vi "Parameter.vi"(9 "In":string, 10 "VIId":string, 11 "VariablesRef":T4) -> ()   [LabVIEW 2018, in "String.lvlib"]
uses:
  String.lvlib
  <userlib>/_OpenG.lib/dictionary/dictionary.llb/Dictionary Object RefNum__ogtk.ctl
  <userlib>/_OpenG.lib/dictionary/dictionary.llb/Dictionary Object RefNum - Enum__ogtk.ctl
  <vilib>/Utility/error.llb/whitespace.ctl
  <vilib>/addons/_JKI.lib/Serialization/JSON/JKI JSON Serialization.lvlib
panel:
  in  "Tab Control":enum32{"Config", "控件"}(tab)
  in  "ArrayType":T1(tab)
  in  "字符串_InitialString":string caption="字符串(可通过${..}调用组合字符串)"
  in  "长度_StringSubset":i32 caption="长度"
  in  "偏移_StringSubset":i32 caption="偏移"
  in  "位置_TrimWhitespace":T2 caption="位置" items=["both", "start of string", "end of string"]
  in  "长度_ReplaceSubstring":i32 caption="长度"
  in  "偏移_ReplaceSubstring":i32 caption="偏移"
  in  "子字符串_ReplaceSubstring":string caption="子字符串(可通过${..}调用组合字符串)"
  in  "IgnoreCase_SearchandReplaceString":bool caption="IgnoreCase"
  in  "ReplaceAll_SearchandReplaceString":bool caption="ReplaceAll"
  in  "替换字符串_SearchandReplaceString":string caption="替换字符串(可通过${..}调用组合字符串)"
  in  "偏移_SearchandReplaceString":i32 caption="偏移"
  in  "搜索字符串_SearchandReplaceString":string caption="搜索字符串(可通过${..}调用组合字符串)"
  in  "偏移_MatchPattern":i32 caption="偏移"
  in  "正则表达式_MatchPattern":string caption="正则表达式(仅支持部分正则)"
  in  "多行_MatchRegularExpression":bool caption="多行"
  in  "忽略大小写_MatchRegularExpression":bool caption="忽略大小写"
  in  "偏移_MatchRegularExpression":i32 caption="偏移"
  in  "正则表达式_MatchRegularExpression":string caption="正则表达式(支持全部正则)"
  in  "UTC格式_FormatDate/TimeString":bool
  in  "时间格式字符串_FormatDate/TimeString":string
  in  "忽略大小写_StartWith":bool caption="忽略大小写"
  in  "子字符串_StartWith":string caption="子字符串(可通过${..}调用组合字符串)"
  in  "子字符串_EndWith":string caption="子字符串(可通过${..}调用组合字符串)"
  in  "忽略大小写_EndWith":bool caption="忽略大小写"
  in  "SubString_AfterSubstring":string caption="子字符串(可通过${..}调用组合字符串)"
  in  "SubString_BeforeSubstring":string caption="子字符串(可通过${..}调用组合字符串)"
  in  "后子字符串_MiddleSubstring":string caption="后子字符串(可通过${..}调用组合字符串)"
  in  "前子字符串_MiddleSubstring":string caption="前子字符串(可通过${..}调用组合字符串)"
  in  "Delimiter_StringTo1DArray":string="\t"
  in  "字符串变量(StringVar)":u16(ring) items=["", "SN", "FileName", "ProductName", "TestLine", "TestStation"]
  in  "方法(Method)":T3(ring)
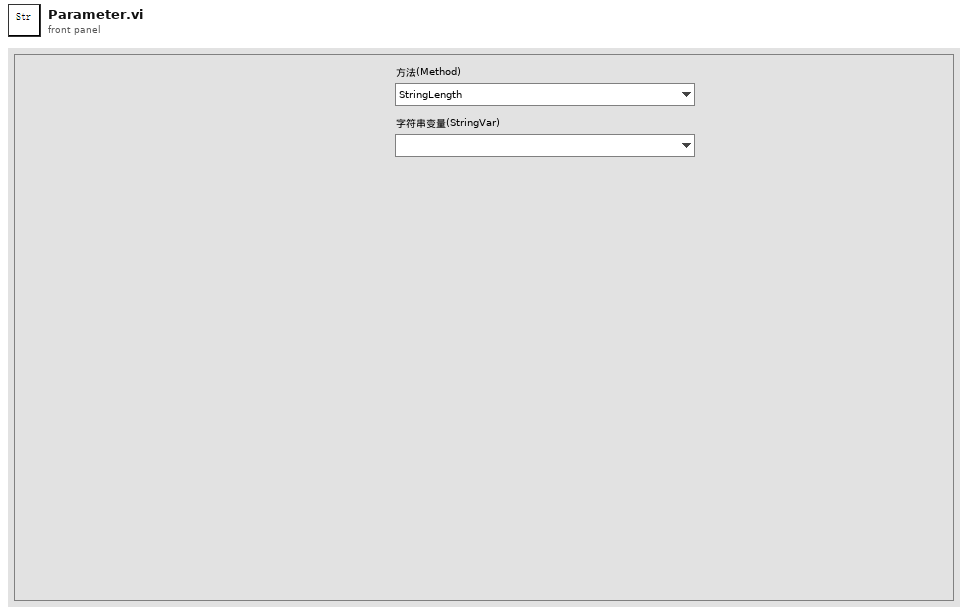
[diagram p1: front panel]
types:
  T1 = enum32{"StringLength", "InitialString", "StringSubset", "TrimWhitespace", "ReplaceSubstring", "SearchandReplaceString", "MatchPattern", "MatchRegularExpression", "FormatDate/TimeString", "ToLowerCase", "ToUpperCase", "StringMD5", "NumStringToHexString", "HexStringToNumString", "StartWith", "EndWith", "AfterSubstring", "BeforeSubstring", "MiddleSubstring", "AsciiToHexString", "HexStringToAscii", "StringTo1DArray", "StringToCharacterArray", "RemoveAllWhitespace"}
  T2 = typedef "whitespace.ctl" = u16
  T3 = enum16{"StringLength", "InitialString", "StringSubset", "TrimWhitespace", "ReplaceSubstring", "SearchandReplaceString", "MatchPattern", "MatchRegularExpression", "FormatDate/TimeString", "ToLowerCase", "ToUpperCase", "StringMD5", "NumStringToHexString", "HexStringToNumString", "StartWith", "EndWith", "AfterSubstring", "BeforeSubstring", "MiddleSubstring", "AsciiToHexString", "HexStringToAscii", "StringTo1DArray", "StringToCharacterArray", "RemoveAllWhitespace"}
  T4 = typedef "Dictionary Object RefNum__ogtk.ctl" = refnum<k1>
  T5 = cluster{"StringLength":cluster{"json":cluster{"Method":string, "StringVar":string}}, "InitialString":cluster{"json":cluster{"Method":string, "Strings":string}}, "StringSubset":cluster{"json":cluster{"Method":string, "StringVar":string, "offset":i32, "length":i32}}, "TrimWhitespace":cluster{"json":cluster{"Method":string, "StringVar":string, "Location":string}}, "ReplaceSubstring":cluster{"json":cluster{"Method":string, "StringVar":string, "Substring":string, "Offset":i32, "Length":i32}}, "SearchandReplaceString":cluster{"json":cluster{"Method":string, "StringVar":string, "SearchString":string, "Offset":i32, "ReplaceString":string, "ReplaceAll":bool, "IgnoreCase":bool}}, "MatchPattern":cluster{"json":cluster{"Method":string, "StringVar":string, "RegularExpression ":string, "Offset":i32}}, "MatchRegularExpression":cluster{"json":cluster{"Method":string, "StringVar":string, "RegularExpression ":string, "Offset":i32, "IgnoreCase":bool, "Multiline":bool}}, "FormatDate/TimeString":cluster{"json":cluster{"Method":string, "TimeFormatString ":string, "UTCFormat":bool}}, "ToLowerCase":cluster{"json":cluster{"Method":string, "StringVar":string}}, "ToUpperCase":cluster{"json":cluster{"Method":string, "StringVar":string}}, "StringMD5":cluster{"json":cluster{"Method":string, "StringVar":string}}, "NumStringToHexString":cluster{"json":cluster{"Method":string, "StringVar":string}}, "HexStringToNumString":cluster{"json":cluster{"Method":string, "StringVar":string}}, "StartWith":cluster{"json":cluster{"Method":string, "StringVar":string, "SubString":string, "IgnoreCasse":bool}}, "EndWith":cluster{"json":cluster{"Method":string, "StringVar":string, "SubString":string, "IgnoreCasse":bool}}, "AfterSubstring":cluster{"json":cluster{"Method":string, "StringVar":string, "SubString":string}}, "BeforeSubstring":cluster{"json":cluster{"Method":string, "StringVar":string, "SubString":string}}, "MiddleSubstring":cluster{"json":cluster{"Method":string, "StringVar":string, "BeforeSubString":string, "AfterSubString":string}}, "AsciiToHexString":cluster{"json":cluster{"Method":string, "StringVar":string}}, "HexStringToAscii":cluster{"json":cluster{"Method":string, "StringVar":string}}, "StringTo1DArray":cluster{"json":cluster{"Method":string, "StringVar":string, "Delimiter":string}}, "StringToCharacterArray":cluster{"json":cluster{"Method":string, "StringVar":string}}, "RemoveAllWhitespace":cluster{"json":cluster{"Method":string, "StringVar":string}}}
  T6 = enum32{"Invalid", "Standard", "Closed", "Hidden", "Minimized", "Maximized"}
  T7 = enum32{"invalid app kind", "Development System", "Run Time System", "Student Edition", "Embedded LabVIEW", "Evaluation", "Custom"}
  T8 = cluster{"Core":cluster{"Current VI Reference":refnum<vi>, "Close Panel on Exit?":bool}, "Parameter":cluster{"VariableRef":T4}, "Synchronize":cluster{"EnqueueData":cluster{"Action":enum16{"Create", "Query", "Revert", "UpdateVariable", "Close"}, "Data":variant}, "Echo":cluster{"VIRef":refnum<vi>, "JsonOut":string, "Status":string}, "Communicate":cluster{"ID":string, "JsonIn":string, "VarRef":T4}, "Queue":refnum<queue>}, "StringClusters":cluster{"StringLength":cluster{"json":cluster{"Method":string, "StringVar":string}}, "InitialString":cluster{"json":cluster{"Method":string, "Strings":string}}, "StringSubset":cluster{"json":cluster{"Method":string, "StringVar":string, "offset":i32, "length":i32}}, "TrimWhitespace":cluster{"json":cluster{"Method":string, "StringVar":string, "Location":string}}, "ReplaceSubstring":cluster{"json":cluster{"Method":string, "StringVar":string, "Substring":string, "Offset":i32, "Length":i32}}, "SearchandReplaceString":cluster{"json":cluster{"Method":string, "StringVar":string, "SearchString":string, "Offset":i32, "ReplaceString":string, "ReplaceAll":bool, "IgnoreCase":bool}}, "MatchPattern":cluster{"json":cluster{"Method":string, "StringVar":string, "RegularExpression ":string, "Offset":i32}}, "MatchRegularExpression":cluster{"json":cluster{"Method":string, "StringVar":string, "RegularExpression ":string, "Offset":i32, "IgnoreCase":bool, "Multiline":bool}}, "FormatDate/TimeString":cluster{"json":cluster{"Method":string, "TimeFormatString ":string, "UTCFormat":bool}}, "ToLowerCase":cluster{"json":cluster{"Method":string, "StringVar":string}}, "ToUpperCase":cluster{"json":cluster{"Method":string, "StringVar":string}}, "StringMD5":cluster{"json":cluster{"Method":string, "StringVar":string}}, "NumStringToHexString":cluster{"json":cluster{"Method":string, "StringVar":string}}, "HexStringToNumString":cluster{"json":cluster{"Method":string, "StringVar":string}}, "StartWith":cluster{"json":cluster{"Method":string, "StringVar":string, "SubString":string, "IgnoreCasse":bool}}, "EndWith":cluster{"json":cluster{"Method":string, "StringVar":string, "SubString":string, "IgnoreCasse":bool}}, "AfterSubstring":cluster{"json":cluster{"Method":string, "StringVar":string, "SubString":string}}, "BeforeSubstring":cluster{"json":cluster{"Method":string, "StringVar":string, "SubString":string}}, "MiddleSubstring":cluster{"json":cluster{"Method":string, "StringVar":string, "BeforeSubString":string, "AfterSubString":string}}, "AsciiToHexString":cluster{"json":cluster{"Method":string, "StringVar":string}}, "HexStringToAscii":cluster{"json":cluster{"Method":string, "StringVar":string}}, "StringTo1DArray":cluster{"json":cluster{"Method":string, "StringVar":string, "Delimiter":string}}, "StringToCharacterArray":cluster{"json":cluster{"Method":string, "StringVar":string}}, "RemoveAllWhitespace":cluster{"json":cluster{"Method":string, "StringVar":string}}}}
  T9 = cluster{"EnqueueData":cluster{"Action":enum16{"Create", "Query", "Revert", "UpdateVariable", "Close"}, "Data":variant}, "Echo":cluster{"VIRef":refnum<vi>, "JsonOut":string, "Status":string}, "Communicate":cluster{"ID":string, "JsonIn":string, "VarRef":T4}, "Queue":refnum<queue>}
  T10 = cluster{"Current VI Reference":refnum<vi>, "Close Panel on Exit?":bool}
  T11 = cluster{"json":cluster{"Method":string, "StringVar":string}}
  T12 = cluster{"json":cluster{"Method":string, "Strings":string}}
  T13 = cluster{"json":cluster{"Method":string, "StringVar":string, "offset":i32, "length":i32}}
  T14 = cluster{"json":cluster{"Method":string, "StringVar":string, "Location":string}}
  T15 = cluster{"json":cluster{"Method":string, "StringVar":string, "Substring":string, "Offset":i32, "Length":i32}}
  T16 = cluster{"json":cluster{"Method":string, "StringVar":string, "SearchString":string, "Offset":i32, "ReplaceString":string, "ReplaceAll":bool, "IgnoreCase":bool}}
  T17 = cluster{"json":cluster{"Method":string, "StringVar":string, "RegularExpression ":string, "Offset":i32}}
  T18 = cluster{"json":cluster{"Method":string, "StringVar":string, "RegularExpression ":string, "Offset":i32, "IgnoreCase":bool, "Multiline":bool}}
  T19 = cluster{"json":cluster{"Method":string, "TimeFormatString ":string, "UTCFormat":bool}}
  T20 = cluster{"json":cluster{"Method":string, "StringVar":string, "SubString":string, "IgnoreCasse":bool}}
  T21 = cluster{"json":cluster{"Method":string, "StringVar":string, "SubString":string}}
  T22 = cluster{"json":cluster{"Method":string, "StringVar":string, "BeforeSubString":string, "AfterSubString":string}}
  T23 = cluster{"json":cluster{"Method":string, "StringVar":string, "Delimiter":string}}
  T24 = cluster{"Action":enum16{"Create", "Query", "Revert", "UpdateVariable", "Close"}, "Data":variant}
  T25 = cluster{"ID":string, "JsonIn":string, "VarRef":T4}
  T26 = enum16{"Create", "Query", "Revert", "UpdateVariable", "Close"}
  T27 = cluster{"VIRef":refnum<vi>, "JsonOut":string, "Status":string}
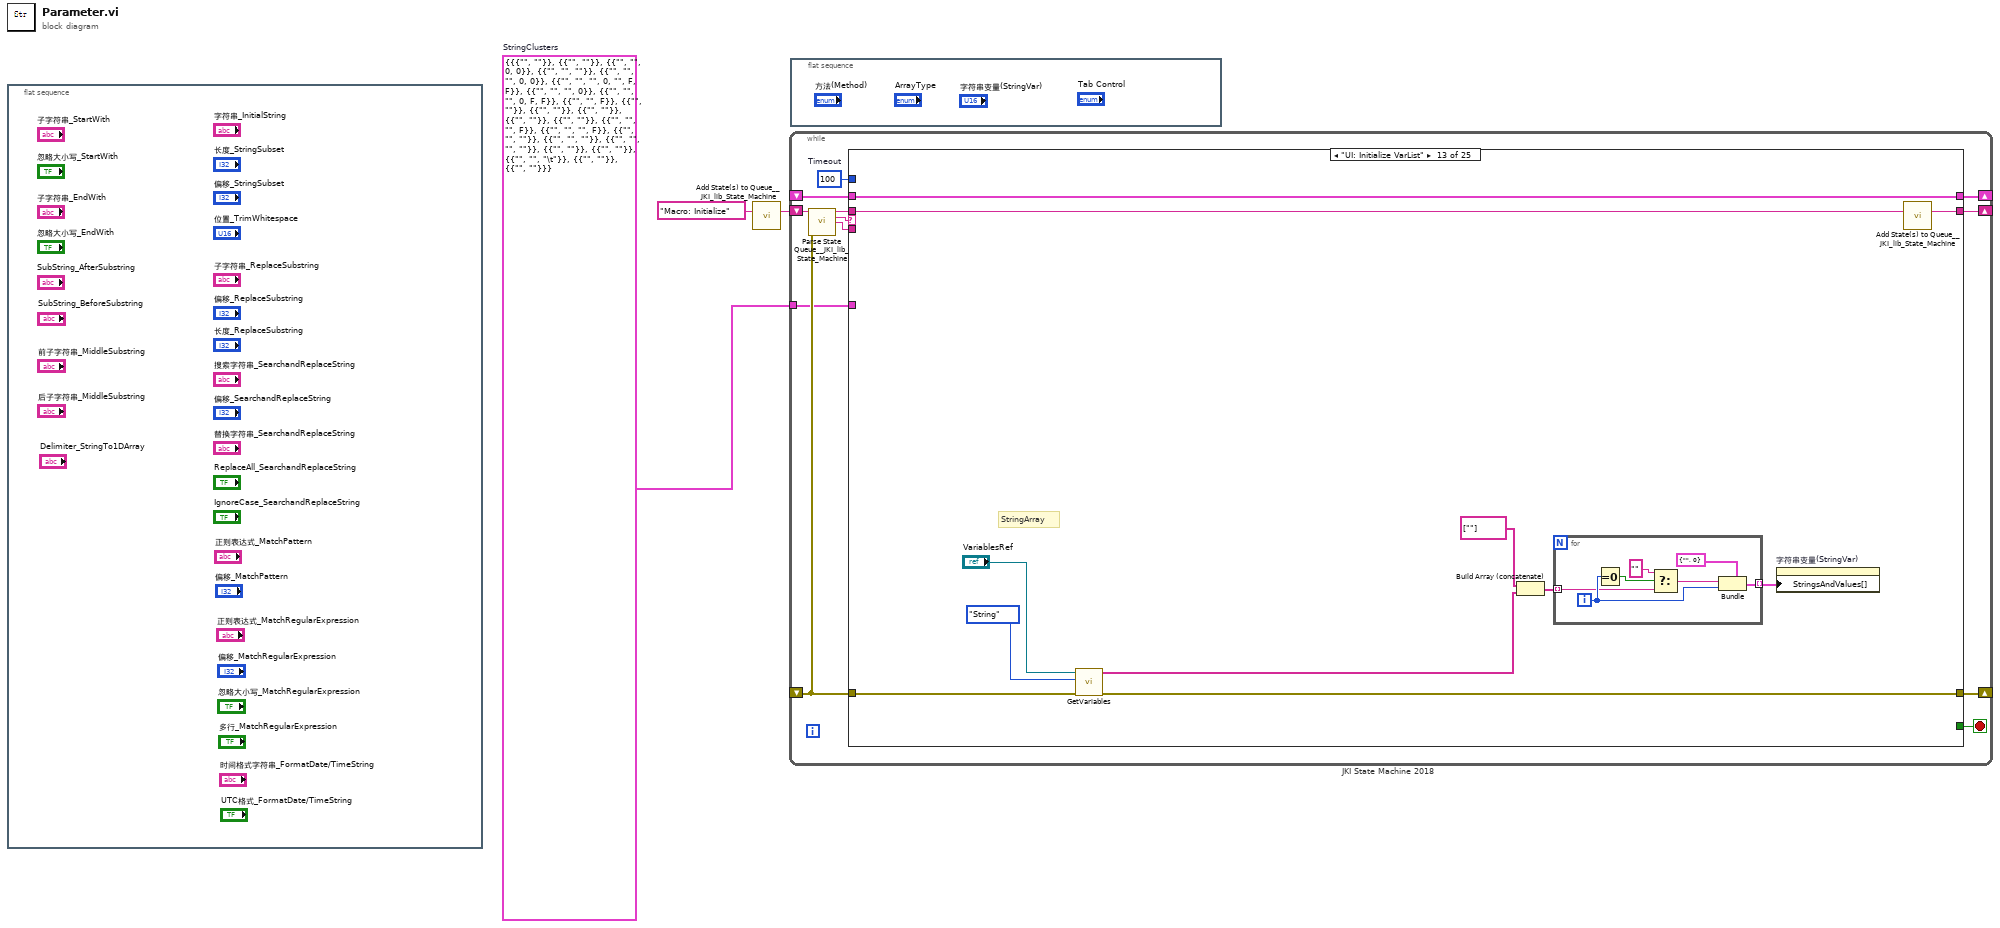
[diagram p0: block diagram]
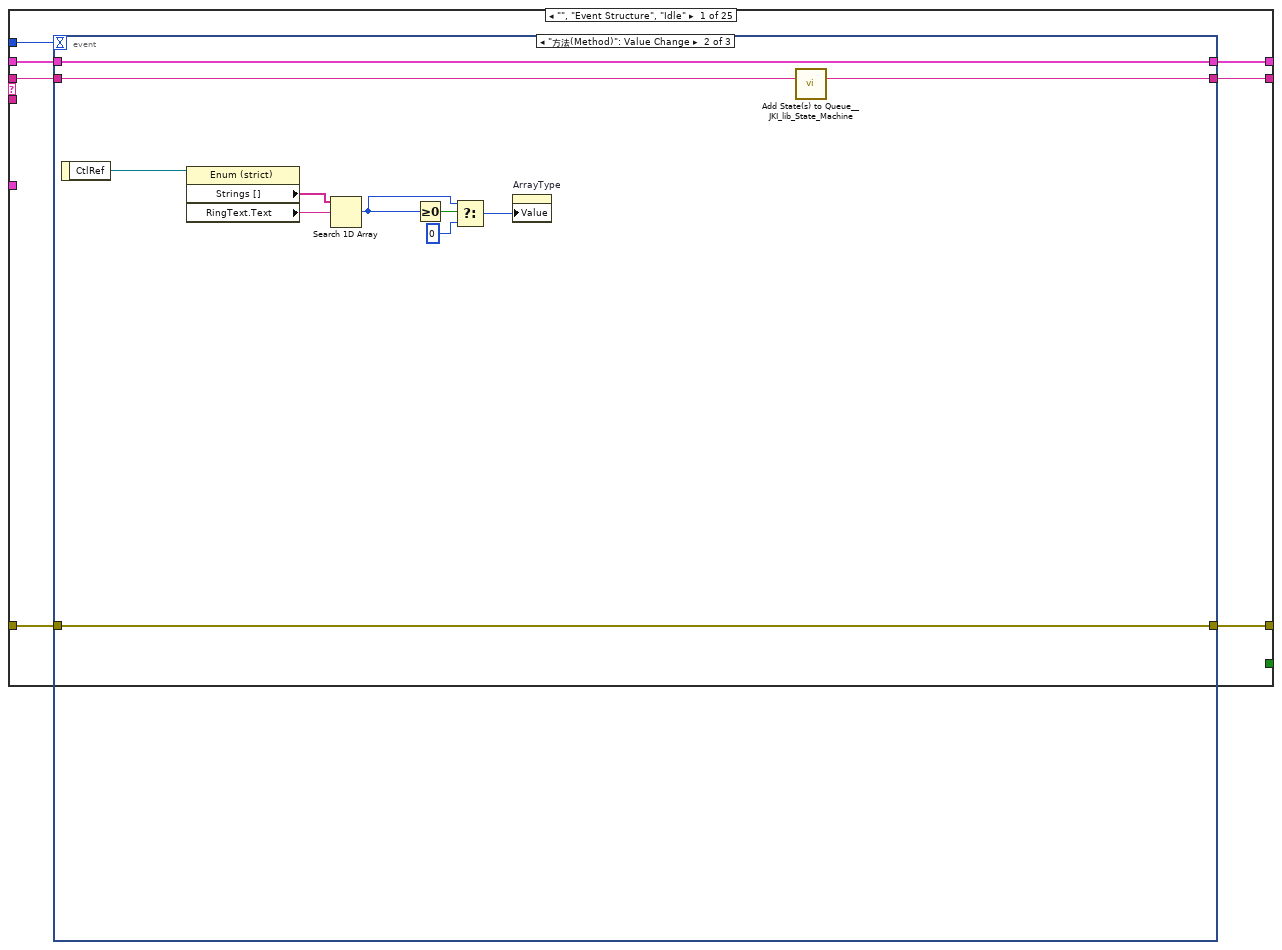
[diagram p2: hidden frame]
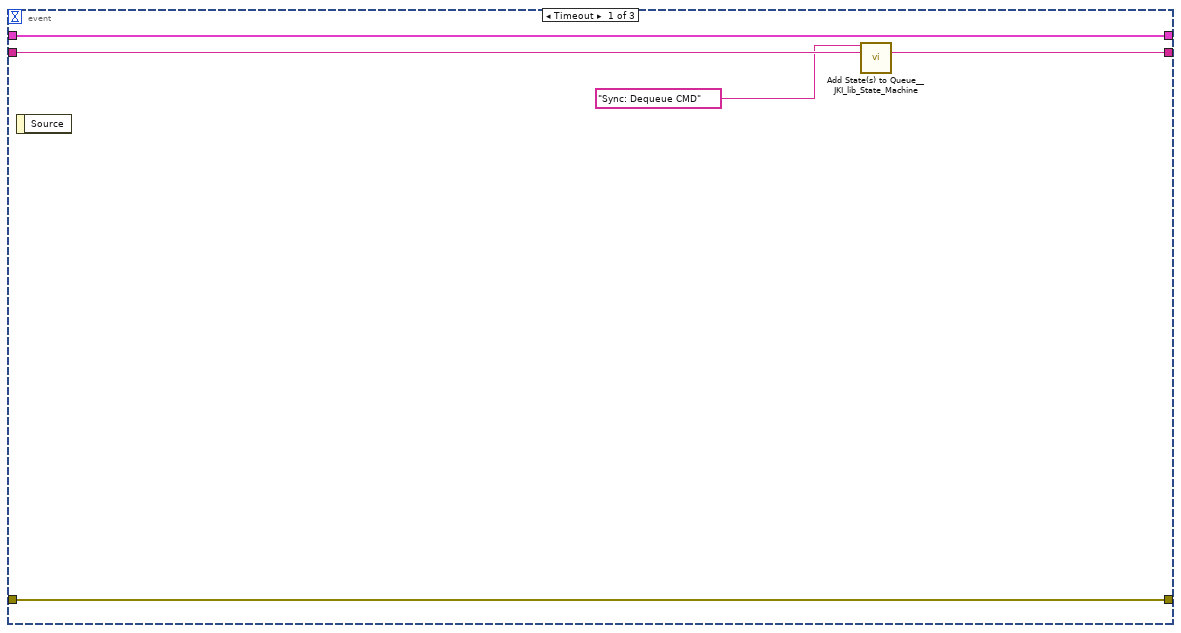
[diagram p3: hidden frame]
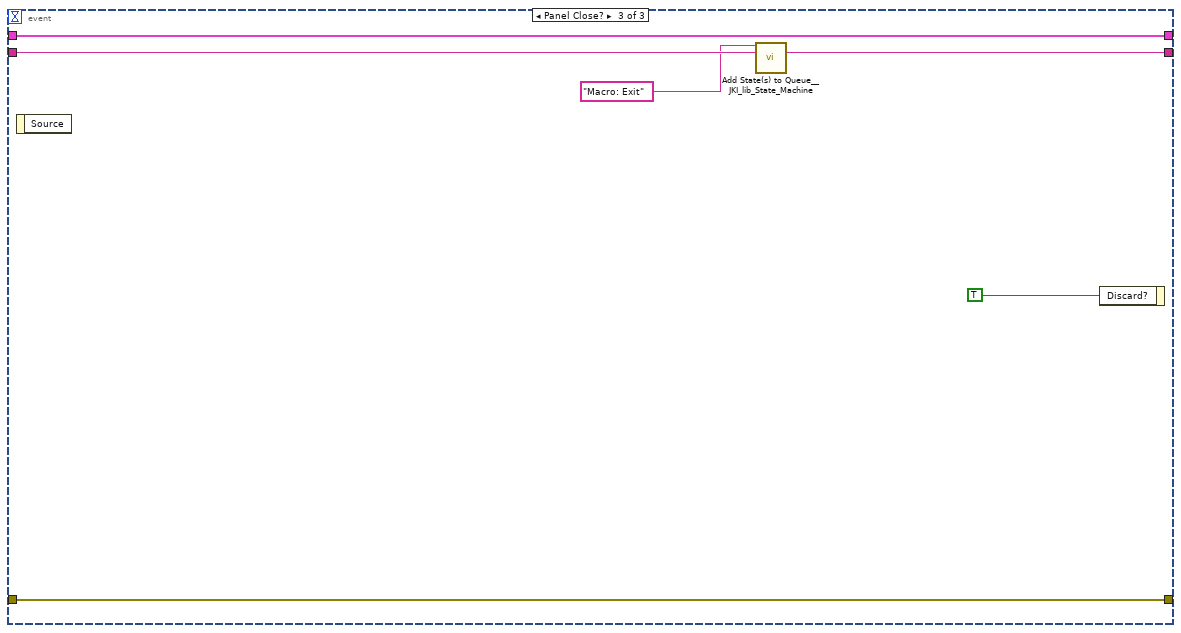
[diagram p4: hidden frame]
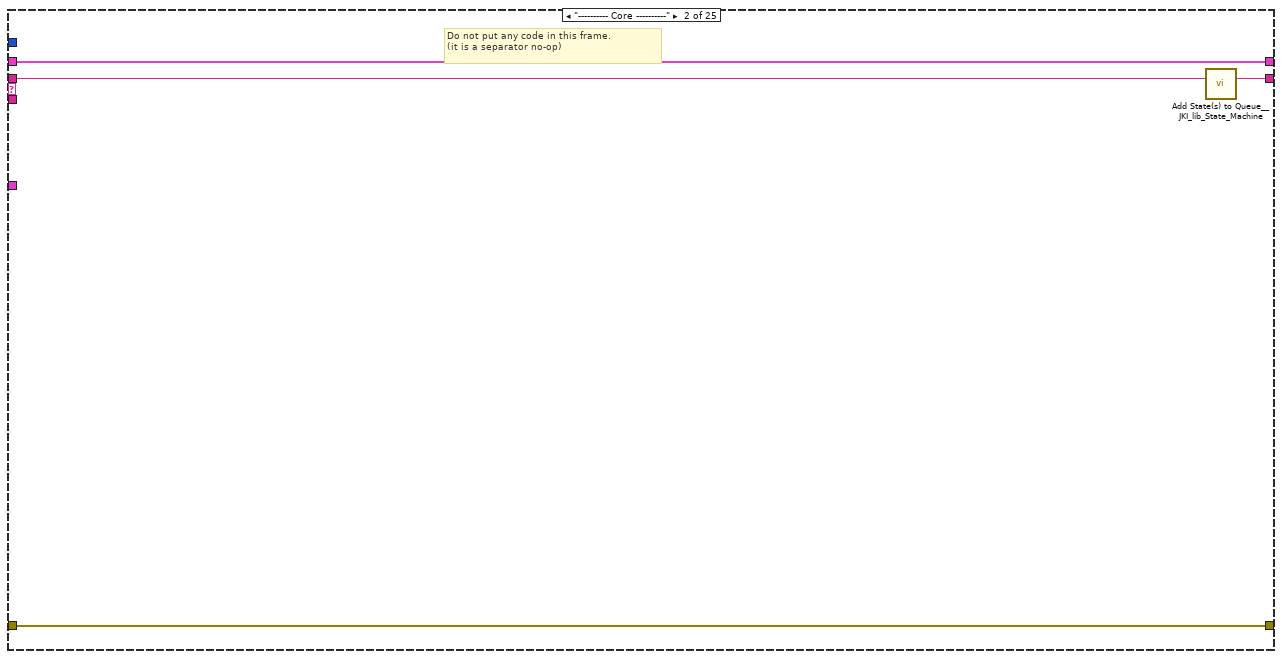
[diagram p5: hidden frame]
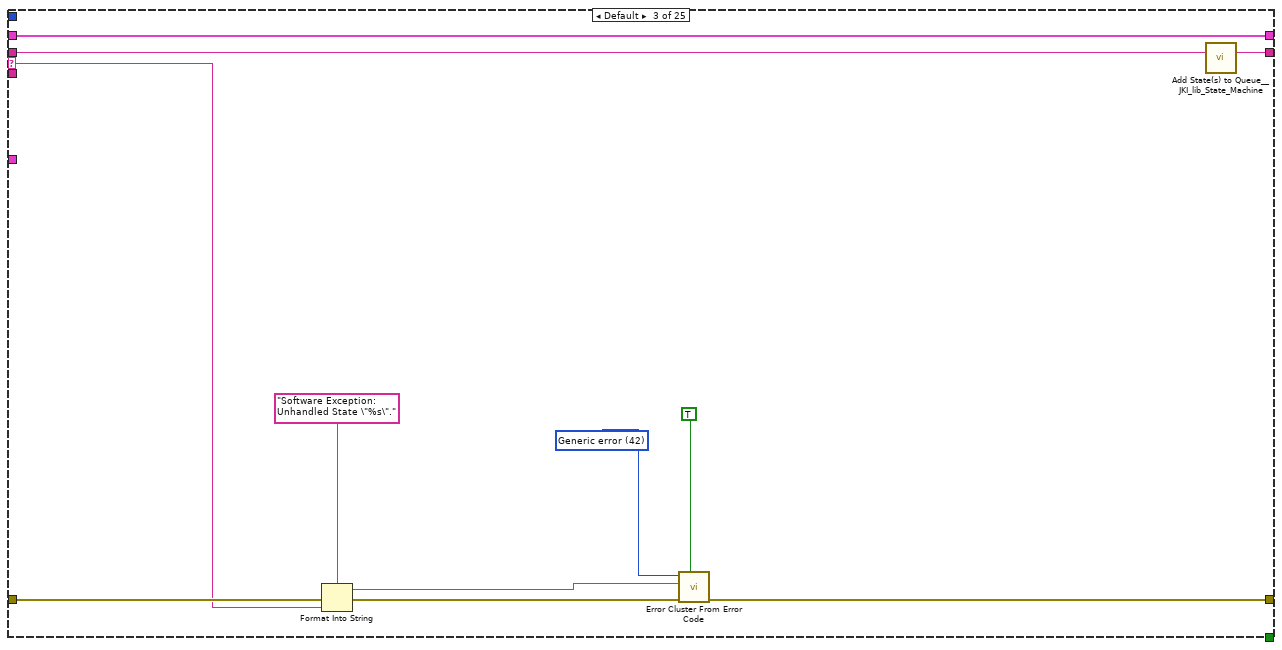
[diagram p6: hidden frame]
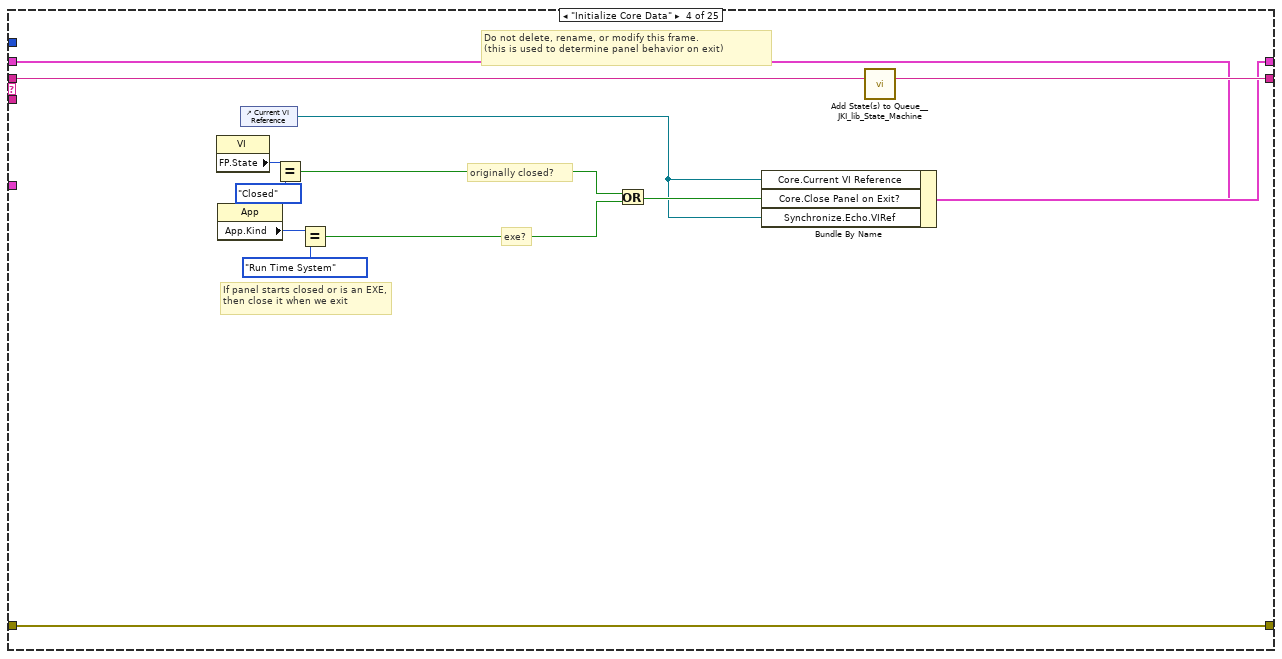
[diagram p7: hidden frame]
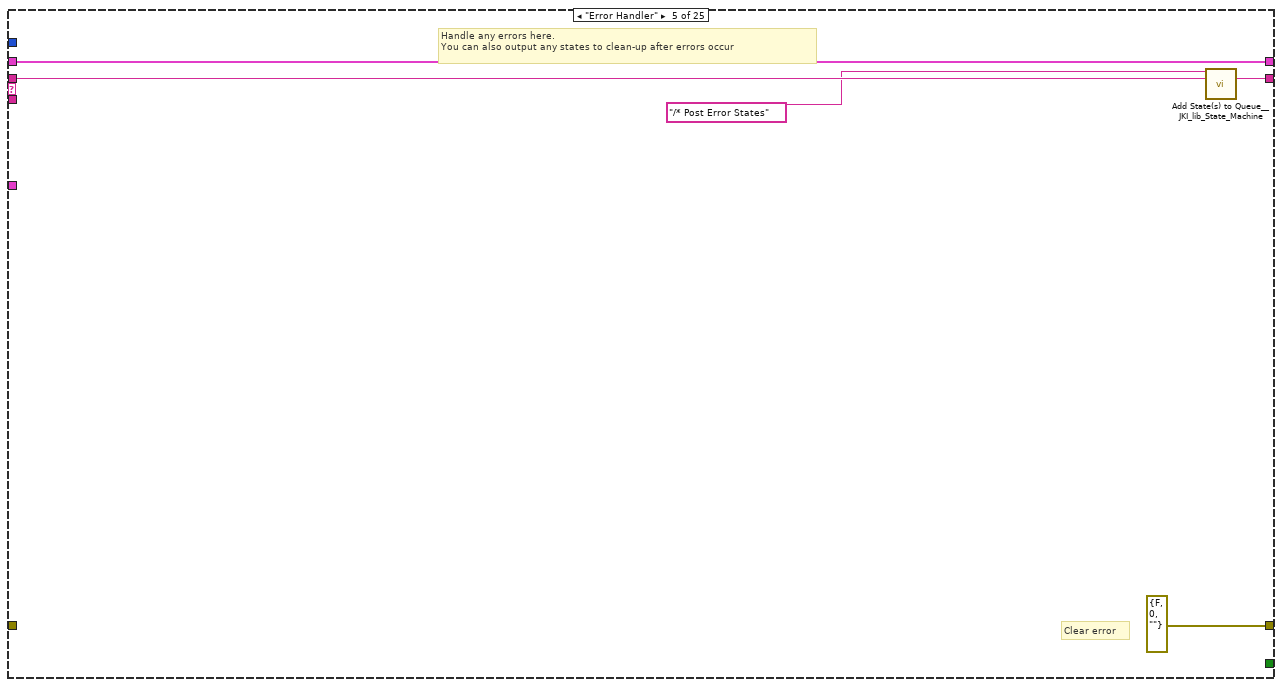
[diagram p8: hidden frame]
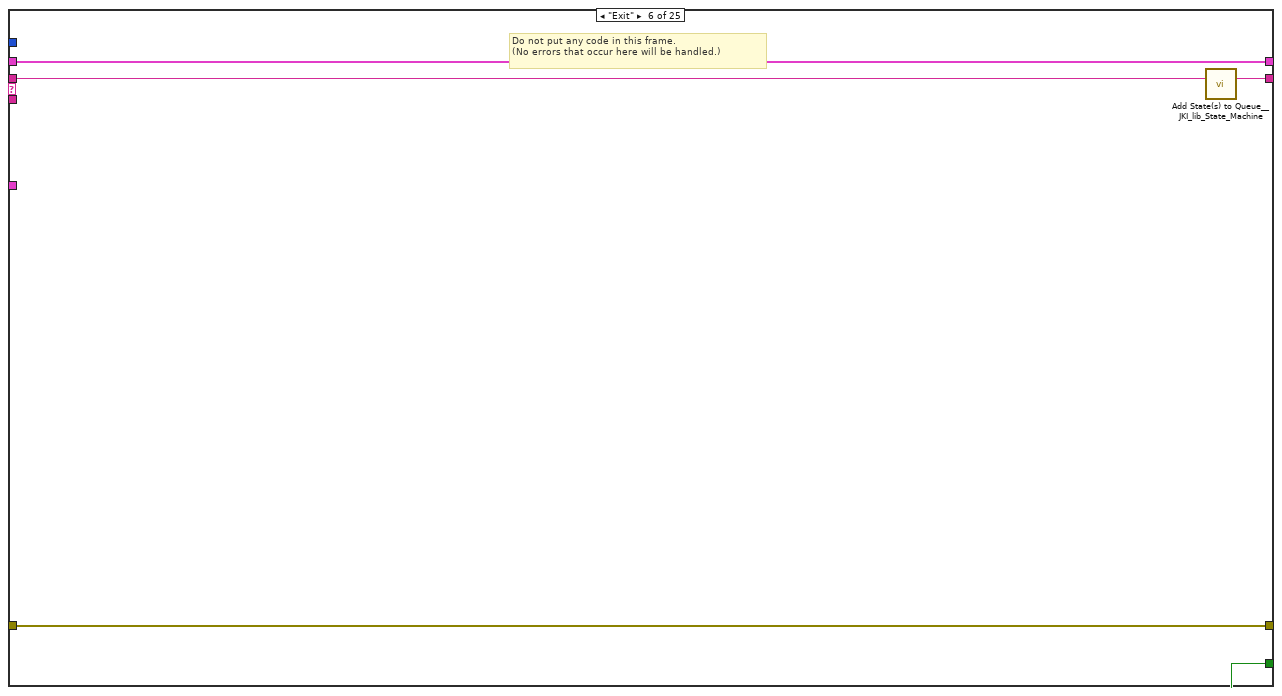
[diagram p9: hidden frame]
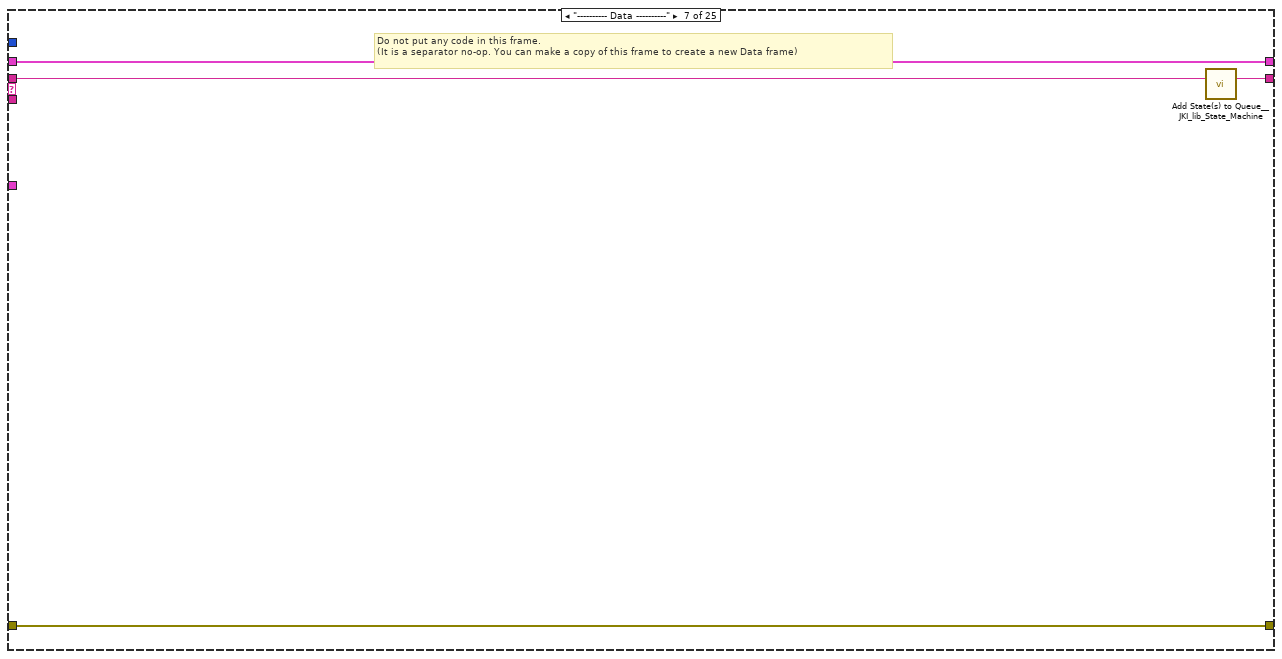
[diagram p10: hidden frame]
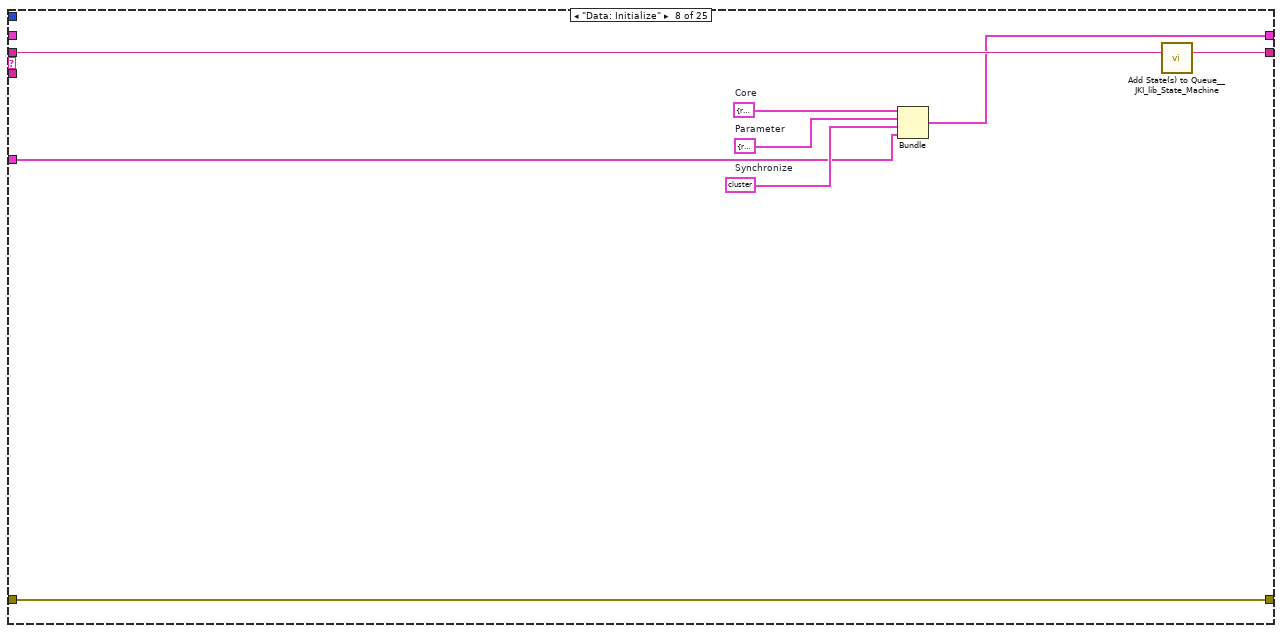
[diagram p11: hidden frame]
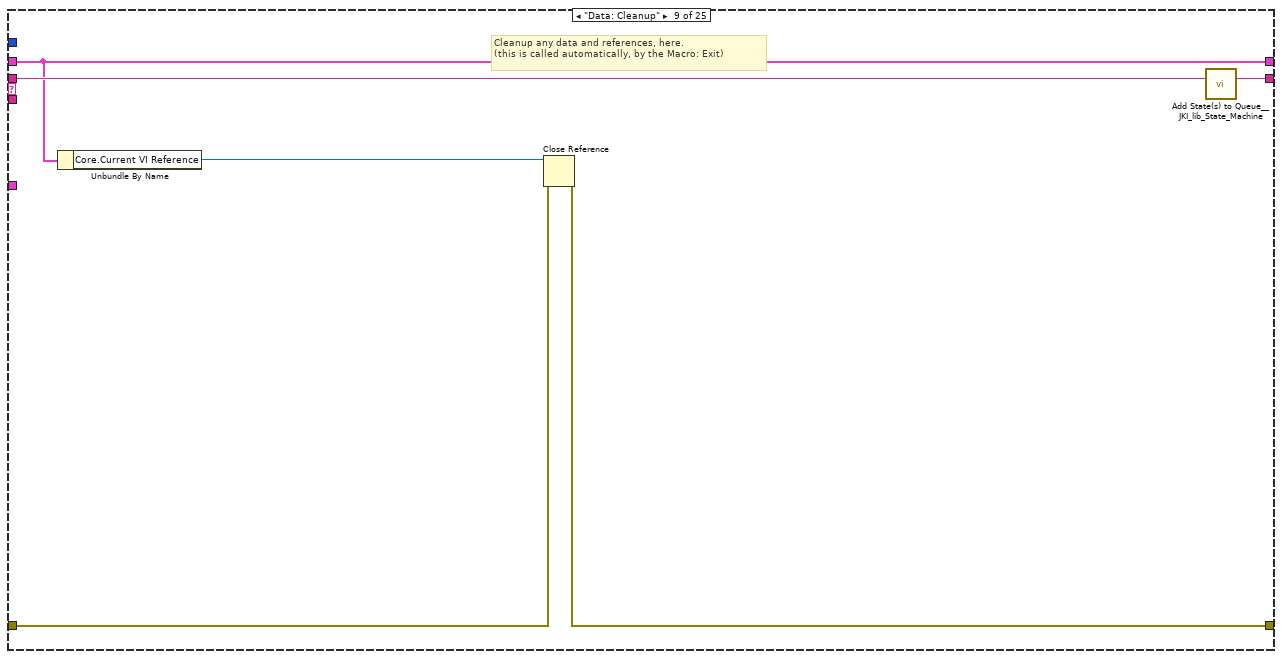
[diagram p12: hidden frame]
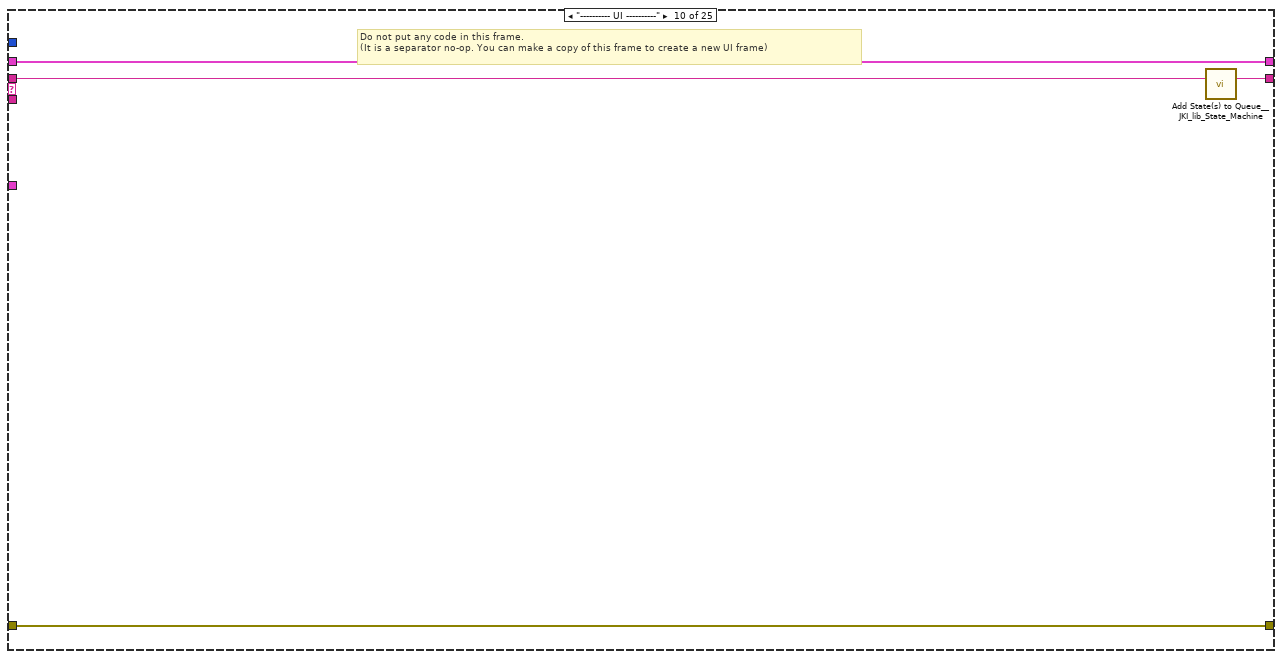
[diagram p13: hidden frame]
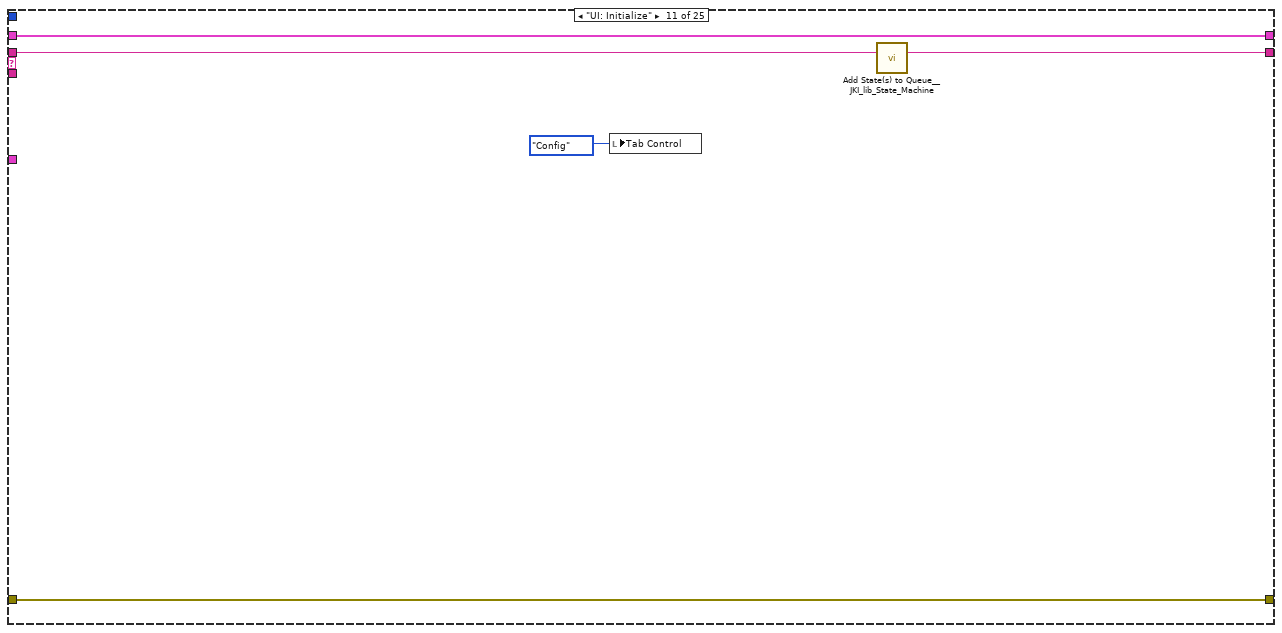
[diagram p14: hidden frame]
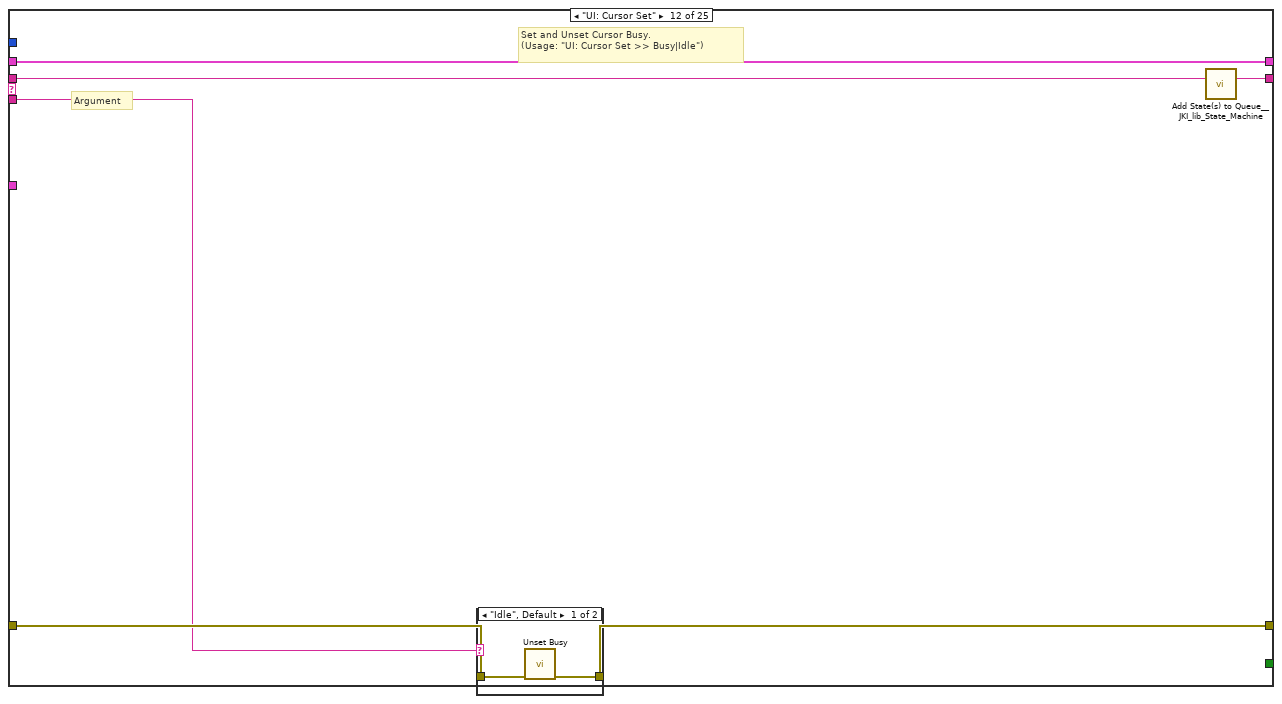
[diagram p15: hidden frame]
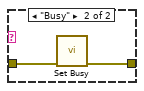
[diagram p16: hidden frame]
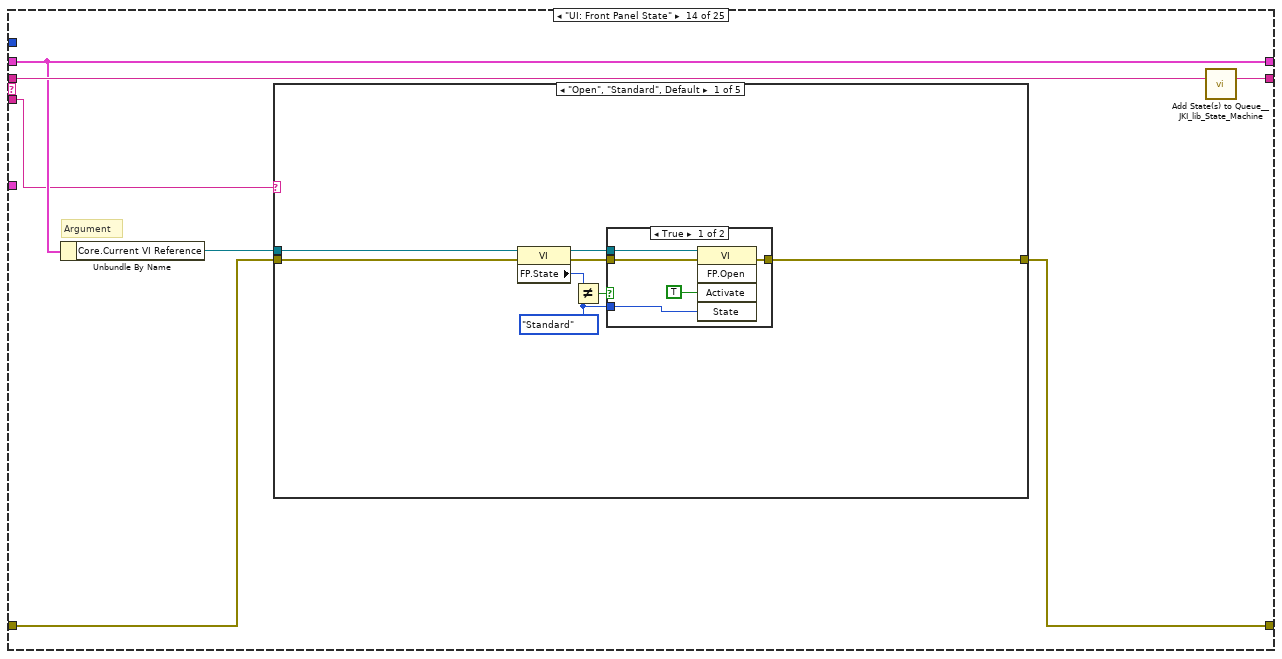
[diagram p17: hidden frame]
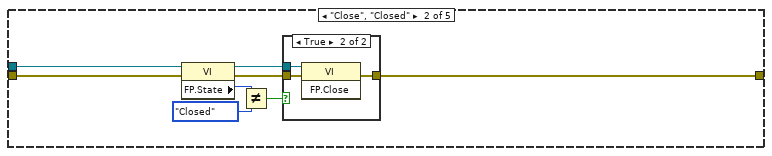
[diagram p19: hidden frame]
diagram:
  w1 = T5 {"StringLength"={"json"={"Method"="", "StringVar"=""}}, "InitialString"={"json"={"Method"="", "Strings"=""}}, "StringSubset"={"json"={"Method"="", "StringVar"="", "offset"=0, "length"=0}}, "TrimWhitespace"={"json"={"Method"="", "StringVar"="", "Location"=""}}, "ReplaceSubstring"={"json"={"Method"="", "StringVar"="", "Substring"="", "Offset"=0, "Length"=0}}, "SearchandReplaceString"={"json"={"Method"="", "StringVar"="", "SearchString"="", "Offset"=0, "ReplaceString"="", "ReplaceAll"=FALSE, "IgnoreCase"=FALSE}}, "MatchPattern"={"json"={"Method"="", "StringVar"="", "RegularExpression "="", "Offset"=0}}, "MatchRegularExpression"={"json"={"Method"="", "StringVar"="", "RegularExpression "="", "Offset"=0, "IgnoreCase"=FALSE, "Multiline"=FALSE}}, "FormatDate/TimeString"={"json"={"Method"="", "TimeFormatString "="", "UTCFormat"=FALSE}}, "ToLowerCase"={"json"={"Method"="", "StringVar"=""}}, "ToUpperCase"={"json"={"Method"="", "StringVar"=""}}, "StringMD5"={"json"={"Method"="", "StringVar"=""}}, "NumStringToHexString"={"json"={"Method"="", "StringVar"=""}}, "HexStringToNumString"={"json"={"Method"="", "StringVar"=""}}, "StartWith"={"json"={"Method"="", "StringVar"="", "SubString"="", "IgnoreCasse"=FALSE}}, "EndWith"={"json"={"Method"="", "StringVar"="", "SubString"="", "IgnoreCasse"=FALSE}}, "AfterSubstring"={"json"={"Method"="", "StringVar"="", "SubString"=""}}, "BeforeSubstring"={"json"={"Method"="", "StringVar"="", "SubString"=""}}, "MiddleSubstring"={"json"={"Method"="", "StringVar"="", "BeforeSubString"="", "AfterSubString"=""}}, "AsciiToHexString"={"json"={"Method"="", "StringVar"=""}}, "HexStringToAscii"={"json"={"Method"="", "StringVar"=""}}, "StringTo1DArray"={"json"={"Method"="", "StringVar"="", "Delimiter"="\t"}}, "StringToCharacterArray"={"json"={"Method"="", "StringVar"=""}}, "RemoveAllWhitespace"={"json"={"Method"="", "StringVar"=""}}}  # StringClusters
  n1 = flat-sequence {
    frame #0 {
    }
  }
  n2 = call <vilib>:"Add State(s) to Queue__JKI_lib_State_Machine.vi"("State(s) in (\"\")"="Macro: Initialize") -> ("States Out"=w3:string)  [unwired: 14 in]
  n3 = while "JKI State Machine 2018" {
    shift-right: [w8] -> _
    shift-left: _ -> [w7]
    shift-right: [w11] -> _
    shift-left: _ -> [w5]
    shift-right: [w10] -> _
    shift-left: w3 -> [w12]
    tunnel: w1 -> [w4]
    stop <- w9 stop-if-true
    w6 = 100  # Timeout
    n4 = call <vilib>:"Parse State Queue__JKI_lib_State_Machine.vi"("State Queue"=w12, "Error In (no error)"=w5) -> ("Remaining States"=w14:string, "Current State"=w15:string, "Arguments"=w13:string)  [unwired: 11 in]
    n5 = case shown="\"UI: Initialize VarList\"" w15 {
      selector: w15 -> [_ _ w49 _ _ _ _ _ _ _ _ _ _ _ _ _ _ _ _ _ _ _ _ _ _]
      tunnel: w14 -> [w22 w48 w53 w72 w77 w82 w86 w94 w100 w104 w109 w115 w130 w144 w213 w218 w228 w232 w240 w647 w895 w904 w919 w963 w978]
      tunnel: w13 -> [_ _ _ _ _ _ _ _ _ _ _ w110 _ w138 _ _ _ _ _ _ _ _ _ _ _]
      tunnel: w7 -> [w20 w45 w51 w65 w74 w80 w83 _ w95 w101 w106 w113 w128 w140 w210 w215 w225 w229 w235 w640 w892 w897 w917 w960 w967]
      tunnel: [w19 w46 w55 w69 errorcluster {"status"=FALSE, "code"=0, "source"=""} ("error out") w79 w84 w92 w96 w102 w105 w111 w127 w141 w211 w216 w226 w230 w236 w644 w893 w901 w906 w958 w965] -> w11
      tunnel: w5 -> [w18 w46 w54 w69 _ w79 w84 w92 w97 w102 w105 w112 w125 w142 w211 w216 w226 w230 w237 w643 w893 w902 w915 w959 w966]
      tunnel: [w21 w47 w52 w71 w76 w81 w85 w93 w99 w103 w108 w114 w129 w143 w212 w217 w227 w231 w239 w646 w894 w903 w918 w962 w977] -> w10
      tunnel: [_ _ _ _ _ TRUE _ _ _ _ _ _ _ _ _ _ _ _ _ _ _ _ _ _ _] -> w9
      tunnel: [w17 w45 w51 w70 w74 w80 w83 w89 w95 w101 w106 w113 w128 w140 w210 w215 w225 w229 w235 w645 w892 w899 w908 w960 w967] -> w8
      tunnel: w6 -> [w16 _ _ _ _ _ _ _ _ _ _ _ _ _ _ _ _ _ _ _ _ _ _ _ _]
      tunnel: w4 -> [_ _ _ _ _ _ _ w87 _ _ _ _ _ _ _ _ _ _ _ _ _ _ _ _ _]
      frame "", "Event Structure", "Idle" {
        n6 = event shown="[1] \"方法(Method)\": Value Change" {
          selector: _ -> [_ _ _]
          dyn-events: _ -> [_ _ _]
          timeout: w16 -> [_ _ _]
          tunnel: w22 -> [w27 w38 w44]
          tunnel: [w26 w37 w43] -> w21
          tunnel: w20 -> [w24 w35 w41]
          tunnel: [w25 w36 w42] -> w19
          tunnel: w18 -> [w25 w36 w42]
          tunnel: [w24 w35 w41] -> w17
          event Timeout {
            n7 = event-data() -> ()  [unwired: 1 in, 1 out]
            n8 = call <vilib>:"Add State(s) to Queue__JKI_lib_State_Machine.vi"("State(s) in Front (\"\")"="Sync: Dequeue CMD" ("State(s) in Front (\"\")"), "State(s) in (\"\")"=w27) -> ("States Out"=w26:string)  [unwired: 13 in]
          }
          event "方法(Method)": Value Change {
            n9 = event-data() -> ("CtlRef"=w31:refnum<vi>)  [unwired: 1 in]
            n10 = property class="Enum (strict)"(reference=w31) -> ("Strings []"=w30:string[], "RingText.Text"=w29:string)  [unwired: 1 in, 2 out]
            n11 = Search 1D Array(1D array=w30, element=w29) -> (index of element=w33:i32)  [unwired: 1 in]
            n12 = Greater Or Equal To 0?(x=w33) -> (x >= 0?=w34:bool)
            n13 = Select(t=w33, s=w34, f=0) -> (s? t:f=w28:i32)
            n14 = property on="ArrayType" class="TabCtl (strict)"("Value"=w28) -> ()  [unwired: 2 in, 2 out]
            n15 = call <vilib>:"Add State(s) to Queue__JKI_lib_State_Machine.vi"("State(s) in (\"\")"=w38) -> ("States Out"=w37:string)  [unwired: 14 in]
          }
          event Panel Close? {
            n16 = event-data() -> ()  [unwired: 1 in, 1 out]
            n17 = call <vilib>:"Add State(s) to Queue__JKI_lib_State_Machine.vi"("State(s) in Front (\"\")"="Macro: Exit", "State(s) in (\"\")"=w44) -> ("States Out"=w43:string)  [unwired: 13 in]
            n18 = event-data("Discard?"=TRUE) -> ()  [unwired: 1 in, 1 out]
          }
        }
      }
      frame "---------- Core ----------" {
        # "Do not put any code in this frame.\n(it is a separator no-op)"
        n19 = call <vilib>:"Add State(s) to Queue__JKI_lib_State_Machine.vi"("State(s) in (\"\")"=w48) -> ("States Out"=w47:string)  [unwired: 14 in]
      }
      frame Default {
        w58 = 42 items=["No error", "Argument error", "Memory is full", "Out of zone", "End of file", "File already open", "Generic file I/O error", "File not found", "File permission error", "Disk is full", "Duplicate path", "Too many files open", "System feature not enabled", "Resource file not found", "Cannot add resource", "Resource not found", "Image not found", "Image memory error", "Pen does not exist", "Config type invalid", "Config token not found", "Config parse error", "Config memory error", "Bad external code format", "Bad external code offset", "External code not present", "Null window", "Destroy window error", "Null menu", "Print aborted", "Bad print record", "Print driver error", "Windows error during printing", "Memory error during printing", "Print dialog error", "Generic print error", "Invalid device refnum", "Device not found", "Device parameter error", "Device unit error", "Cannot open device", "Device call aborted", "Generic error", "Cancelled by user", "Object ID too low", "Object ID too high", "Object not in heap", "Unknown heap", "Unknown object (invalid DefProc)", "Unknown object (DefProc not in table)", "Message out of range", "Invalid (null) method", "Unknown message", "Manager call not supported", "Bad address", "Network operation in progress", "Network operation timed out", "Connection is busy", "Network attribute not supported", "Network error", "Address in use", "System out of memory", "Connection aborted", "Connection refused", "Not connected", "Already connected", "Connection closed", "Initialization error (interapplication manager)", "Bad occurrence", "Wait on unbound occurrence handler", "Occurrence queue overflow", "Datalog type conflict", "Unused", "Unrecognized type (interapplication manager)", "Memory corrupt", "Failed to make temporary DLL", "Old CIN version", "Drag socket not found", "Failed to load drop-object", "Failed to register OLE object", "Failed to release OLE object", "Format specifier type mismatch", "Unknown format specifier", "Too few format specifiers", "Too many format specifiers", "Scan failed", "Newer CIN version", "Error converting to variant", "Runtime menu error", "Password tampered", "Variant attribute not found", "Incompatible variant data type", "Event data is not available", "Event Store is not present", "Occurrence is not found", "Event Queue is not created", "Event info is not available", "Refnum passed is NULL", "Error retrieving Class GUID", "Error retrieving CoClass GUID", "Error retrieving TypeLib GUID.", "Bad built application magic bytes.", "Specific driver is different from the specific driver associated with the Logical Name.", "There is no session opened to the class driver.", "Max Error", "MAX - Error with config objects", "MAX - Error loading configuration", "MAX - Group not supported"]
        n20 = Format Into String(format string="Software Exception: Unhandled State \"%s\"." ("message"), error in=w54, w49) -> (resulting string=w57:string, error out=w56:errorcluster)  [unwired: 1 in]
        n21 = call <vilib>:"Error Cluster From Error Code.vi"("show call chain? (False)"=TRUE, "error in (no error)"=w56, "error message (\"\")"=w57, "error code (0)"=w58) -> ("error out"=w55:errorcluster)  [unwired: 5 in]
        n22 = call <vilib>:"Add State(s) to Queue__JKI_lib_State_Machine.vi"("State(s) in (\"\")"=w53) -> ("States Out"=w52:string)  [unwired: 14 in]
      }
      frame "Initialize Core Data" {
        # "Do not delete, rename, or modify this frame.\n(this is used to determine panel behavior on exit)"
        # "originally closed?"
        # "exe?"
        # "If panel starts closed or is an EXE, then close it when we exit"
        n23 = property class="VI"() -> ("FP.State"=w63:T6)  [unwired: 2 in, 2 out]
        n24 = property class="App"() -> ("App.Kind"=w68:T7)  [unwired: 2 in, 2 out]
        n25 = control-ref of="Current VI Reference"() -> (w60:refnum<vi>)
        n26 = Equal?(x=w63, y=T6."Closed" ("Front Panel Window:State")) -> (x = y?=w61:bool)
        n27 = Equal?(x=w68, y=T7."Run Time System" ("Application:Kind")) -> (x = y?=w66:bool)
        n28 = Or(x=w61, y=w66) -> (x .or. y?=w64:bool)
        n29 = Bundle By Name(cluster=w65, "Core.Current VI Reference"=w60, "Core.Close Panel on Exit?"=w64, "Synchronize.Echo.VIRef"=w60) -> (w70:T8)
        n30 = call <vilib>:"Add State(s) to Queue__JKI_lib_State_Machine.vi"("State(s) in (\"\")"=w72) -> ("States Out"=w71:string)  [unwired: 14 in]
      }
      frame "Error Handler" {
        # "Handle any errors here.\nYou can also output any states to clean-up after errors occur"
        # "Clear error"
        n31 = call <vilib>:"Add State(s) to Queue__JKI_lib_State_Machine.vi"("State(s) in Front (\"\")"="/* Post Error States", "State(s) in (\"\")"=w77) -> ("States Out"=w76:string)  [unwired: 13 in]
      }
      frame "Exit" {
        # "Do not put any code in this frame.\n(No errors that occur here will be handled.)"
        n32 = call <vilib>:"Add State(s) to Queue__JKI_lib_State_Machine.vi"("State(s) in (\"\")"=w82) -> ("States Out"=w81:string)  [unwired: 14 in]
      }
      frame "---------- Data ----------" {
        # "Do not put any code in this frame.\n(It is a separator no-op. You can make a copy of this frame to create a new Data frame)"
        n33 = call <vilib>:"Add State(s) to Queue__JKI_lib_State_Machine.vi"("State(s) in (\"\")"=w86) -> ("States Out"=w85:string)  [unwired: 14 in]
      }
      frame "Data: Initialize" {
        w88 = cluster{"VariableRef":T4} {"VariableRef"=refnum}  # Parameter
        w90 = T9 {"EnqueueData"={"Action"=enum."Create", "Data"=variant}, "Echo"={"VIRef"=refnum, "JsonOut"="", "Status"=""}, "Communicate"={"ID"="", "JsonIn"="", "VarRef"=refnum}, "Queue"=refnum}  # Synchronize
        w91 = T10 {"Current VI Reference"=refnum, "Close Panel on Exit?"=FALSE}  # Core
        n34 = Bundle("Core"=w91, "Parameter"=w88, "Synchronize"=w90, "StringClusters"=w87) -> (w89:T8)  [unwired: 1 in]
        n35 = call <vilib>:"Add State(s) to Queue__JKI_lib_State_Machine.vi"("State(s) in (\"\")"=w94) -> ("States Out"=w93:string)  [unwired: 14 in]
      }
      frame "Data: Cleanup" {
        # "Cleanup any data and references, here.\n(this is called automatically, by the Macro: Exit)"
        n36 = Unbundle By Name(w95) -> ("Core.Current VI Reference"=w98:refnum<vi>)
        n37 = Close Reference(reference=w98, error in (no error)=w97) -> (error out=w96:errorcluster)
        n38 = call <vilib>:"Add State(s) to Queue__JKI_lib_State_Machine.vi"("State(s) in (\"\")"=w100) -> ("States Out"=w99:string)  [unwired: 14 in]
      }
      frame "---------- UI ----------" {
        # "Do not put any code in this frame.\n(It is a separator no-op. You can make a copy of this frame to create a new UI frame)"
        n39 = call <vilib>:"Add State(s) to Queue__JKI_lib_State_Machine.vi"("State(s) in (\"\")"=w104) -> ("States Out"=w103:string)  [unwired: 14 in]
      }
      frame "UI: Initialize" {
        n40 = local write "Tab Control"(enum32{"Config", "控件"}."Config" ("Tab Control")) -> ()
        n41 = call <vilib>:"Add State(s) to Queue__JKI_lib_State_Machine.vi"("State(s) in (\"\")"=w109) -> ("States Out"=w108:string)  [unwired: 14 in]
      }
      frame "UI: Cursor Set" {
        # "Argument"
        # "Set and Unset Cursor Busy.\n(Usage: \"UI: Cursor Set >> Busy|Idle\")"
        n42 = case shown="\"Idle\", Default" w110 {
          tunnel: w112 -> [w117 w119]
          tunnel: [w116 w118] -> w111
          frame "Idle", Default {
            n43 = call <vilib>:"Unset Busy.vi"("error in (no error)"=w117) -> ("error out"=w116:errorcluster)  [unwired: 10 in]
          }
          frame "Busy" {
            n44 = call <vilib>:"Set Busy.vi"("error in (no error)"=w119) -> ("error out"=w118:errorcluster)  [unwired: 9 in, 1 out]
          }
        }
        n45 = call <vilib>:"Add State(s) to Queue__JKI_lib_State_Machine.vi"("State(s) in (\"\")"=w115) -> ("States Out"=w114:string)  [unwired: 14 in]
      }
      frame "UI: Initialize VarList" {
        # "StringArray"
        n46 = call "GetVariables.vi"("error in (no error)"=w125, "VariableType"=enum16{"String", "StringArray"}."String", "DicRef"="VariablesRef") -> ("error out"=w127:errorcluster, "VariableArray"=w120:string[])  [unwired: 7 in]
        n47 = Build Array (concatenate)(string[] [""] ("array"), w120) -> (w123:string[])
        n48 = for {
          tunnel: [w136] -> w121 mode=indexing
          tunnel: w123 -> [w131] mode=indexing
          i -> [w135]
          n49 = Equal To 0?(x=w135) -> (x = 0?=w134:bool)
          n50 = Select(t="", s=w134, f=w131) -> (s? t:f=w133:string)
          n51 = Bundle(cluster=cluster{"String":string, "Value":u16} {"String"="", "Value"=0}, "String"=w133, "Value"=w135) -> (w136:cluster{"String":string, "Value":u16})
        }
        n52 = property on="字符串变量(StringVar)" class="Ring (strict)"("StringsAndValues[]"=w121) -> ()  [unwired: 2 in, 2 out]
        n53 = call <vilib>:"Add State(s) to Queue__JKI_lib_State_Machine.vi"("State(s) in (\"\")"=w130) -> ("States Out"=w129:string)  [unwired: 14 in]
      }
      frame "UI: Front Panel State" {
        # "Argument"
        n54 = Unbundle By Name(w140) -> ("Core.Current VI Reference"=w139:refnum<vi>)
        n55 = case shown="\"Open\", \"Standard\", Default" w138 {
          tunnel: w142 -> [w150 w165 w176 w189 w202]
          tunnel: [w152 w166 w178 w191 w204] -> w141
          tunnel: w139 -> [w151 w163 w177 w190 w203]
          frame "Open", "Standard", Default {
            w145 = T6."Standard" ("State")
            n56 = property class="VI"(reference=w151, error in=w150) -> (reference out=w148:refnum<vi>, error out=w149:errorcluster, "FP.State"=w147:T6)
            n57 = Not Equal?(x=w147, y=w145) -> (x != y?=w146:bool)
            n58 = case shown="True" w146 {
              tunnel: [w156 w158] -> w152
              tunnel: w149 -> [w155 w158]
              tunnel: w148 -> [w154 _]
              tunnel: w145 -> [w153 _]
              frame True {
                n59 = invoke class="VI" method="FP.Open"(reference=w154, error in=w155, "Activate"=TRUE, "State"=w153) -> (error out=w156:errorcluster)  [unwired: 1 in, 4 out]
              }
              frame False {
              }
            }
          }
          frame "Close", "Closed" {
            n60 = property class="VI"(reference=w163, error in=w165) -> (reference out=w162:refnum<vi>, error out=w164:errorcluster, "FP.State"=w160:T6)
            n61 = Not Equal?(x=w160, y=T6."Closed" ("Front Panel Window:State")) -> (x != y?=w159:bool)
            n62 = case shown="True" w159 {
              tunnel: [w167 w170] -> w166
              tunnel: w164 -> [w167 w169]
              tunnel: w162 -> [_ w168]
              frame False {
              }
              frame True {
                n63 = invoke class="VI" method="FP.Close"(reference=w168, error in=w169) -> (error out=w170:errorcluster)  [unwired: 1 in, 2 out]
              }
            }
          }
          frame "Hidden", "Hide" {
            w171 = T6."Hidden" ("State")
            n64 = property class="VI"(reference=w177, error in=w176) -> (reference out=w174:refnum<vi>, error out=w175:errorcluster, "FP.State"=w173:T6)
            n65 = Not Equal?(x=w173, y=w171) -> (x != y?=w172:bool)
            n66 = case shown="True" w172 {
              tunnel: [w182 w183] -> w178
              tunnel: w175 -> [w181 w183]
              tunnel: w174 -> [w180 _]
              tunnel: w171 -> [w179 _]
              frame True {
                n67 = invoke class="VI" method="FP.Open"(reference=w180, error in=w181, "State"=w179) -> (error out=w182:errorcluster)  [unwired: 2 in, 4 out]
              }
              frame False {
              }
            }
          }
          frame "Minimize", "Minimized" {
            w184 = T6."Minimized" ("State")
            n68 = property class="VI"(reference=w190, error in=w189) -> (reference out=w187:refnum<vi>, error out=w188:errorcluster, "FP.State"=w186:T6)
            n69 = Not Equal?(x=w186, y=w184) -> (x != y?=w185:bool)
            n70 = case shown="True" w185 {
              tunnel: [w195 w196] -> w191
              tunnel: w188 -> [w194 w196]
              tunnel: w187 -> [w193 _]
              tunnel: w184 -> [w192 _]
              frame True {
                n71 = invoke class="VI" method="FP.Open"(reference=w193, error in=w194, "State"=w192) -> (error out=w195:errorcluster)  [unwired: 2 in, 4 out]
              }
              frame False {
              }
            }
          }
          frame "Maximize", "Maximized" {
            w197 = T6."Maximized" ("State")
            n72 = property class="VI"(reference=w203, error in=w202) -> (reference out=w200:refnum<vi>, error out=w201:errorcluster, "FP.State"=w199:T6)
            n73 = Not Equal?(x=w199, y=w197) -> (x != y?=w198:bool)
            n74 = case shown="True" w198 {
              tunnel: [w208 w209] -> w204
              tunnel: w201 -> [w207 w209]
              tunnel: w200 -> [w206 _]
              tunnel: w197 -> [w205 _]
              frame True {
                n75 = invoke class="VI" method="FP.Open"(reference=w206, error in=w207, "State"=w205) -> (error out=w208:errorcluster)  [unwired: 2 in, 4 out]
              }
              frame False {
              }
            }
          }
        }
        n76 = call <vilib>:"Add State(s) to Queue__JKI_lib_State_Machine.vi"("State(s) in (\"\")"=w144) -> ("States Out"=w143:string)  [unwired: 14 in]
      }
      frame "---------- Macro ----------" {
        n77 = call <vilib>:"Add State(s) to Queue__JKI_lib_State_Machine.vi"("State(s) in (\"\")"=w213) -> ("States Out"=w212:string)  [unwired: 14 in]
      }
      frame "Macro: Initialize" {
        n78 = call <vilib>:"Add State(s) to Queue__JKI_lib_State_Machine.vi"("State(s) in Front (\"\")"="Data: Initialize\nInitialize Core Data\nUI: Initialize\nSync: Obtain CMD Queue\nSync: Dequeue CMD\nUI: Initialize VarList\nParameter: Parse Parameter", "State(s) in (\"\")"=w218) -> ("States Out"=w217:string)  [unwired: 13 in]
      }
      frame "Macro: Exit" {
        n79 = Unbundle By Name(w225) -> ("Core.Close Panel on Exit?"=w224:bool)
        n80 = Select(t="UI: Front Panel State >> Close", s=w224, f="") -> (s? t:f=w221:string)
        n81 = call <vilib>:"Add State(s) to Queue__JKI_lib_State_Machine.vi"("State(s) in (\"\")"=w221, "State(s) at Back (\"\")"="Sync: Release CMD Queue\nData: Cleanup\nExit") -> ("States Out"=w219:string)  [unwired: 13 in]
        n82 = call <vilib>:"Add State(s) to Queue__JKI_lib_State_Machine.vi"("State(s) in Front (\"\")"=w219, "State(s) in (\"\")"=w228) -> ("States Out"=w227:string)  [unwired: 13 in]
      }
      frame "---------- Parameter ----------" {
        # "Template Separator\n(You can make a copy of, or modify, this frame)"
        n83 = call <vilib>:"Add State(s) to Queue__JKI_lib_State_Machine.vi"("State(s) in (\"\")"=w232) -> ("States Out"=w231:string)  [unwired: 14 in]
      }
      frame "Parameter: Parse Parameter" {
        n84 = Unbundle By Name(w235) -> ("StringClusters"=w234:T5)
        n85 = Empty String/Path?(string/path="In") -> (empty?=w238:bool)
        n86 = case shown="False" w238 {
          tunnel: "In" -> [w249 _]
          tunnel: w237 -> [w254 w638]
          tunnel: [w253 w638] -> w236
          tunnel: w234 -> [w252 _]
          frame False {
            n87 = Match Pattern(string=w249, regular expression="\"Method\":\"") -> (after substring=w248:string)  [unwired: 1 in, 3 out]
            n88 = Match Pattern(string=w248, regular expression="\",") -> (before substring=w247:string)  [unwired: 1 in, 3 out]
            n89 = case shown="\"StringTo1DArray\"" w247 {
              tunnel: w249 -> [w267 w277 w294 w315 w333 w353 w370 w389 w400 w415 w430 w445 w460 w475 w492 w509 w525 w541 w558 w573 w588 w604 w619 w634 _]
              tunnel: w254 -> [w265 w275 w292 w313 w331 w351 w368 w387 w398 w413 w428 w443 w458 w473 w490 w507 w523 w539 w556 w571 w586 w602 w617 w632 w637]
              tunnel: [w264 w274 w291 w312 w330 w350 w367 w386 w397 w412 w427 w442 w457 w472 w489 w506 w522 w538 w555 w570 w585 w601 w616 w631 w637] -> w253
              tunnel: w252 -> [w256 w272 w289 w310 w328 w348 w365 w384 w395 w410 w425 w440 w455 w470 w487 w504 w520 w536 w553 w568 w583 w599 w614 w629 _]
              tunnel: [w257 w273 w290 w311 w329 w349 w366 w385 w396 w411 w426 w441 w456 w471 w488 w505 w521 w537 w554 w569 w584 w600 w615 w630 _] -> w242
              frame "StringLength" {
                n90 = Unbundle By Name(w256) -> ("StringLength"=w255:T11)
                n91 = call <vilib>:"Unflatten From JSON String.vi"("Type and Defaults"=w255, "error in (no error)"=w265, "JSON String"=w267) -> ("error out"=w268:errorcluster, "Variant"=w269:variant)  [unwired: 7 in]
                n92 = Variant To Data(error in=w268, type=w255, Variant=w269) -> (data=w266:T11, error out=w264:errorcluster)
                n93 = Unbundle By Name(w266) -> ("json.Method"=w257:string, "json.StringVar"=w259:string)
                n94 = property on="字符串变量(StringVar)" class="Ring (strict)"() -> ("Strings []"=w260:string[])  [unwired: 2 in, 2 out]
                n95 = Search 1D Array(1D array=w260, element=w259) -> (index of element=w262:i32)  [unwired: 1 in]
                n96 = Greater Or Equal To 0?(x=w262) -> (x >= 0?=w261:bool)
                n97 = Select(t=w262, s=w261, f=0) -> (s? t:f=w258:i32)
                n98 = property on="字符串变量(StringVar)" class="Ring (strict)"("Value"=w258) -> ()  [unwired: 2 in, 2 out]
              }
              frame "InitialString" {
                n99 = Unbundle By Name(w272) -> ("InitialString"=w271:T12)
                n100 = call <vilib>:"Unflatten From JSON String.vi"("Type and Defaults"=w271, "error in (no error)"=w275, "JSON String"=w277) -> ("error out"=w278:errorcluster, "Variant"=w279:variant)  [unwired: 7 in]
                n101 = Variant To Data(error in=w278, type=w271, Variant=w279) -> (data=w276:T12, error out=w274:errorcluster)
                n102 = Unbundle By Name(w276) -> ("json.Method"=w273:string, "json.Strings"=w270:string)
                n103 = local write "字符串_InitialString"(w270) -> ()
              }
              frame "StringSubset" {
                n104 = Unbundle By Name(w289) -> ("StringSubset"=w288:T13)
                n105 = call <vilib>:"Unflatten From JSON String.vi"("Type and Defaults"=w288, "error in (no error)"=w292, "JSON String"=w294) -> ("error out"=w295:errorcluster, "Variant"=w296:variant)  [unwired: 7 in]
                n106 = Variant To Data(error in=w295, type=w288, Variant=w296) -> (data=w293:T13, error out=w291:errorcluster)
                n107 = Unbundle By Name(w293) -> ("json.Method"=w290:string, "json.StringVar"=w282:string, "json.offset"=w281:i32, "json.length"=w280:i32)
                n108 = local write "偏移_StringSubset"(w281) -> ()
                n109 = local write "长度_StringSubset"(w280) -> ()
                n110 = property on="字符串变量(StringVar)" class="Ring (strict)"() -> ("Strings []"=w285:string[])  [unwired: 2 in, 2 out]
                n111 = Search 1D Array(1D array=w285, element=w282) -> (index of element=w287:i32)  [unwired: 1 in]
                n112 = Greater Or Equal To 0?(x=w287) -> (x >= 0?=w286:bool)
                n113 = Select(t=w287, s=w286, f=0) -> (s? t:f=w284:i32)
                n114 = property on="字符串变量(StringVar)" class="Ring (strict)"("Value"=w284) -> ()  [unwired: 2 in, 2 out]
              }
              frame "TrimWhitespace" {
                n115 = Unbundle By Name(w310) -> ("TrimWhitespace"=w309:T14)
                n116 = call <vilib>:"Unflatten From JSON String.vi"("Type and Defaults"=w309, "error in (no error)"=w313, "JSON String"=w315) -> ("error out"=w316:errorcluster, "Variant"=w317:variant)  [unwired: 7 in]
                n117 = Variant To Data(error in=w316, type=w309, Variant=w317) -> (data=w314:T14, error out=w312:errorcluster)
                n118 = Unbundle By Name(w314) -> ("json.Method"=w311:string, "json.StringVar"=w303:string, "json.Location"=w299:string)
                n119 = property on="位置_TrimWhitespace" class="Ring (strict)"() -> ("Strings []"=w300:string[])  [unwired: 2 in, 2 out]
                n120 = property on="字符串变量(StringVar)" class="Ring (strict)"() -> ("Strings []"=w306:string[])  [unwired: 2 in, 2 out]
                n121 = Search 1D Array(1D array=w300, element=w299) -> (index of element=w298:i32)  [unwired: 1 in]
                n122 = Search 1D Array(1D array=w306, element=w303) -> (index of element=w308:i32)  [unwired: 1 in]
                n123 = Greater Or Equal To 0?(x=w298) -> (x >= 0?=w302:bool)
                n124 = Greater Or Equal To 0?(x=w308) -> (x >= 0?=w307:bool)
                n125 = Select(t=w298, s=w302, f=0) -> (s? t:f=w297:i32)
                n126 = Select(t=w308, s=w307, f=0) -> (s? t:f=w305:i32)
                n127 = property on="字符串变量(StringVar)" class="Ring (strict)"("Value"=w305) -> ()  [unwired: 2 in, 2 out]
                n128 = property on="位置_TrimWhitespace" class="Ring (strict)"("Value"=w297) -> ()  [unwired: 2 in, 2 out]
              }
              frame "ReplaceSubstring" {
                n129 = Unbundle By Name(w328) -> ("ReplaceSubstring"=w327:T15)
                n130 = call <vilib>:"Unflatten From JSON String.vi"("Type and Defaults"=w327, "error in (no error)"=w331, "JSON String"=w333) -> ("error out"=w334:errorcluster, "Variant"=w335:variant)  [unwired: 7 in]
                n131 = Variant To Data(error in=w334, type=w327, Variant=w335) -> (data=w332:T15, error out=w330:errorcluster)
                n132 = Unbundle By Name(w332) -> ("json.Method"=w329:string, "json.StringVar"=w321:string, "json.Substring"=w320:string, "json.Offset"=w319:i32, "json.Length"=w318:i32)
                n133 = property on="字符串变量(StringVar)" class="Ring (strict)"() -> ("Strings []"=w324:string[])  [unwired: 2 in, 2 out]
                n134 = local write "子字符串_ReplaceSubstring"(w320) -> ()
                n135 = local write "偏移_ReplaceSubstring"(w319) -> ()
                n136 = local write "长度_ReplaceSubstring"(w318) -> ()
                n137 = Search 1D Array(1D array=w324, element=w321) -> (index of element=w326:i32)  [unwired: 1 in]
                n138 = Greater Or Equal To 0?(x=w326) -> (x >= 0?=w325:bool)
                n139 = Select(t=w326, s=w325, f=0) -> (s? t:f=w323:i32)
                n140 = property on="字符串变量(StringVar)" class="Ring (strict)"("Value"=w323) -> ()  [unwired: 2 in, 2 out]
              }
              frame "SearchandReplaceString" {
                n141 = Unbundle By Name(w348) -> ("SearchandReplaceString"=w347:T16)
                n142 = call <vilib>:"Unflatten From JSON String.vi"("Type and Defaults"=w347, "error in (no error)"=w351, "JSON String"=w353) -> ("error out"=w354:errorcluster, "Variant"=w355:variant)  [unwired: 7 in]
                n143 = Variant To Data(error in=w354, type=w347, Variant=w355) -> (data=w352:T16, error out=w350:errorcluster)
                n144 = Unbundle By Name(w352) -> ("json.Method"=w349:string, "json.StringVar"=w341:string, "json.SearchString"=w340:string, "json.Offset"=w339:i32, "json.ReplaceString"=w338:string, "json.ReplaceAll"=w337:bool, "json.IgnoreCase"=w336:bool)
                n145 = property on="字符串变量(StringVar)" class="Ring (strict)"() -> ("Strings []"=w344:string[])  [unwired: 2 in, 2 out]
                n146 = local write "搜索字符串_SearchandReplaceString"(w340) -> ()
                n147 = local write "ReplaceAll_SearchandReplaceString"(w337) -> ()
                n148 = local write "偏移_SearchandReplaceString"(w339) -> ()
                n149 = local write "替换字符串_SearchandReplaceString"(w338) -> ()
                n150 = local write "IgnoreCase_SearchandReplaceString"(w336) -> ()
                n151 = Search 1D Array(1D array=w344, element=w341) -> (index of element=w346:i32)  [unwired: 1 in]
                n152 = Greater Or Equal To 0?(x=w346) -> (x >= 0?=w345:bool)
                n153 = Select(t=w346, s=w345, f=0) -> (s? t:f=w343:i32)
                n154 = property on="字符串变量(StringVar)" class="Ring (strict)"("Value"=w343) -> ()  [unwired: 2 in, 2 out]
              }
              frame "MatchPattern" {
                n155 = Unbundle By Name(w365) -> ("MatchPattern"=w364:T17)
                n156 = call <vilib>:"Unflatten From JSON String.vi"("Type and Defaults"=w364, "error in (no error)"=w368, "JSON String"=w370) -> ("error out"=w371:errorcluster, "Variant"=w372:variant)  [unwired: 7 in]
                n157 = Variant To Data(error in=w371, type=w364, Variant=w372) -> (data=w369:T17, error out=w367:errorcluster)
                n158 = Unbundle By Name(w369) -> ("json.Method"=w366:string, "json.StringVar"=w358:string, "json.RegularExpression"=w357:string, "json.Offset"=w356:i32)
                n159 = property on="字符串变量(StringVar)" class="Ring (strict)"() -> ("Strings []"=w361:string[])  [unwired: 2 in, 2 out]
                n160 = local write "正则表达式_MatchPattern"(w357) -> ()
                n161 = local write "偏移_MatchPattern"(w356) -> ()
                n162 = Search 1D Array(1D array=w361, element=w358) -> (index of element=w363:i32)  [unwired: 1 in]
                n163 = Greater Or Equal To 0?(x=w363) -> (x >= 0?=w362:bool)
                n164 = Select(t=w363, s=w362, f=0) -> (s? t:f=w360:i32)
                n165 = property on="字符串变量(StringVar)" class="Ring (strict)"("Value"=w360) -> ()  [unwired: 2 in, 2 out]
              }
              frame "MatchRegularExpression" {
                n166 = Unbundle By Name(w384) -> ("MatchRegularExpression"=w383:T18)
                n167 = call <vilib>:"Unflatten From JSON String.vi"("Type and Defaults"=w383, "error in (no error)"=w387, "JSON String"=w389) -> ("error out"=w390:errorcluster, "Variant"=w391:variant)  [unwired: 7 in]
                n168 = Variant To Data(error in=w390, type=w383, Variant=w391) -> (data=w388:T18, error out=w386:errorcluster)
                n169 = Unbundle By Name(w388) -> ("json.Method"=w385:string, "json.StringVar"=w377:string, "json.RegularExpression"=w376:string, "json.Offset"=w375:i32, "json.IgnoreCase"=w374:bool, "json.Multiline"=w373:bool)
                n170 = property on="字符串变量(StringVar)" class="Ring (strict)"() -> ("Strings []"=w380:string[])  [unwired: 2 in, 2 out]
                n171 = local write "正则表达式_MatchRegularExpression"(w376) -> ()
                n172 = local write "偏移_MatchRegularExpression"(w375) -> ()
                n173 = local write "忽略大小写_MatchRegularExpression"(w374) -> ()
                n174 = local write "多行_MatchRegularExpression"(w373) -> ()
                n175 = Search 1D Array(1D array=w380, element=w377) -> (index of element=w382:i32)  [unwired: 1 in]
                n176 = Greater Or Equal To 0?(x=w382) -> (x >= 0?=w381:bool)
                n177 = Select(t=w382, s=w381, f=0) -> (s? t:f=w379:i32)
                n178 = property on="字符串变量(StringVar)" class="Ring (strict)"("Value"=w379) -> ()  [unwired: 2 in, 2 out]
              }
              frame "FormatDate/TimeString" {
                n179 = Unbundle By Name(w395) -> ("FormatDate/TimeString"=w394:T19)
                n180 = call <vilib>:"Unflatten From JSON String.vi"("Type and Defaults"=w394, "error in (no error)"=w398, "JSON String"=w400) -> ("error out"=w401:errorcluster, "Variant"=w402:variant)  [unwired: 7 in]
                n181 = Variant To Data(error in=w401, type=w394, Variant=w402) -> (data=w399:T19, error out=w397:errorcluster)
                n182 = Unbundle By Name(w399) -> ("json.Method"=w396:string, "json.TimeFormatString"=w393:string, "json.UTCFormat"=w392:bool)
                n183 = local write "时间格式字符串_FormatDate/TimeString"(w393) -> ()
                n184 = local write "UTC格式_FormatDate/TimeString"(w392) -> ()
              }
              frame "ToLowerCase" {
                n185 = Unbundle By Name(w410) -> ("ToLowerCase"=w409:T11)
                n186 = call <vilib>:"Unflatten From JSON String.vi"("Type and Defaults"=w409, "error in (no error)"=w413, "JSON String"=w415) -> ("error out"=w416:errorcluster, "Variant"=w417:variant)  [unwired: 7 in]
                n187 = Variant To Data(error in=w416, type=w409, Variant=w417) -> (data=w414:T11, error out=w412:errorcluster)
                n188 = Unbundle By Name(w414) -> ("json.Method"=w411:string, "json.StringVar"=w403:string)
                n189 = property on="字符串变量(StringVar)" class="Ring (strict)"() -> ("Strings []"=w406:string[])  [unwired: 2 in, 2 out]
                n190 = Search 1D Array(1D array=w406, element=w403) -> (index of element=w408:i32)  [unwired: 1 in]
                n191 = Greater Or Equal To 0?(x=w408) -> (x >= 0?=w407:bool)
                n192 = Select(t=w408, s=w407, f=0) -> (s? t:f=w405:i32)
                n193 = property on="字符串变量(StringVar)" class="Ring (strict)"("Value"=w405) -> ()  [unwired: 2 in, 2 out]
              }
              frame "ToUpperCase" {
                n194 = Unbundle By Name(w425) -> ("ToUpperCase"=w424:T11)
                n195 = call <vilib>:"Unflatten From JSON String.vi"("Type and Defaults"=w424, "error in (no error)"=w428, "JSON String"=w430) -> ("error out"=w431:errorcluster, "Variant"=w432:variant)  [unwired: 7 in]
                n196 = Variant To Data(error in=w431, type=w424, Variant=w432) -> (data=w429:T11, error out=w427:errorcluster)
                n197 = Unbundle By Name(w429) -> ("json.Method"=w426:string, "json.StringVar"=w418:string)
                n198 = property on="字符串变量(StringVar)" class="Ring (strict)"() -> ("Strings []"=w421:string[])  [unwired: 2 in, 2 out]
                n199 = Search 1D Array(1D array=w421, element=w418) -> (index of element=w423:i32)  [unwired: 1 in]
                n200 = Greater Or Equal To 0?(x=w423) -> (x >= 0?=w422:bool)
                n201 = Select(t=w423, s=w422, f=0) -> (s? t:f=w420:i32)
                n202 = property on="字符串变量(StringVar)" class="Ring (strict)"("Value"=w420) -> ()  [unwired: 2 in, 2 out]
              }
              frame "StringMD5" {
                n203 = Unbundle By Name(w440) -> ("StringMD5"=w439:T11)
                n204 = call <vilib>:"Unflatten From JSON String.vi"("Type and Defaults"=w439, "error in (no error)"=w443, "JSON String"=w445) -> ("error out"=w446:errorcluster, "Variant"=w447:variant)  [unwired: 7 in]
                n205 = Variant To Data(error in=w446, type=w439, Variant=w447) -> (data=w444:T11, error out=w442:errorcluster)
                n206 = Unbundle By Name(w444) -> ("json.Method"=w441:string, "json.StringVar"=w433:string)
                n207 = property on="字符串变量(StringVar)" class="Ring (strict)"() -> ("Strings []"=w436:string[])  [unwired: 2 in, 2 out]
                n208 = Search 1D Array(1D array=w436, element=w433) -> (index of element=w438:i32)  [unwired: 1 in]
                n209 = Greater Or Equal To 0?(x=w438) -> (x >= 0?=w437:bool)
                n210 = Select(t=w438, s=w437, f=0) -> (s? t:f=w435:i32)
                n211 = property on="字符串变量(StringVar)" class="Ring (strict)"("Value"=w435) -> ()  [unwired: 2 in, 2 out]
              }
              frame "NumStringToHexString" {
                n212 = Unbundle By Name(w455) -> ("NumStringToHexString"=w454:T11)
                n213 = call <vilib>:"Unflatten From JSON String.vi"("Type and Defaults"=w454, "error in (no error)"=w458, "JSON String"=w460) -> ("error out"=w461:errorcluster, "Variant"=w462:variant)  [unwired: 7 in]
                n214 = Variant To Data(error in=w461, type=w454, Variant=w462) -> (data=w459:T11, error out=w457:errorcluster)
                n215 = Unbundle By Name(w459) -> ("json.Method"=w456:string, "json.StringVar"=w448:string)
                n216 = property on="字符串变量(StringVar)" class="Ring (strict)"() -> ("Strings []"=w451:string[])  [unwired: 2 in, 2 out]
                n217 = Search 1D Array(1D array=w451, element=w448) -> (index of element=w453:i32)  [unwired: 1 in]
                n218 = Greater Or Equal To 0?(x=w453) -> (x >= 0?=w452:bool)
                n219 = Select(t=w453, s=w452, f=0) -> (s? t:f=w450:i32)
                n220 = property on="字符串变量(StringVar)" class="Ring (strict)"("Value"=w450) -> ()  [unwired: 2 in, 2 out]
              }
              frame "HexStringToNumString" {
                n221 = Unbundle By Name(w470) -> ("HexStringToNumString"=w469:T11)
                n222 = call <vilib>:"Unflatten From JSON String.vi"("Type and Defaults"=w469, "error in (no error)"=w473, "JSON String"=w475) -> ("error out"=w476:errorcluster, "Variant"=w477:variant)  [unwired: 7 in]
                n223 = Variant To Data(error in=w476, type=w469, Variant=w477) -> (data=w474:T11, error out=w472:errorcluster)
                n224 = Unbundle By Name(w474) -> ("json.Method"=w471:string, "json.StringVar"=w463:string)
                n225 = property on="字符串变量(StringVar)" class="Ring (strict)"() -> ("Strings []"=w466:string[])  [unwired: 2 in, 2 out]
                n226 = Search 1D Array(1D array=w466, element=w463) -> (index of element=w468:i32)  [unwired: 1 in]
                n227 = Greater Or Equal To 0?(x=w468) -> (x >= 0?=w467:bool)
                n228 = Select(t=w468, s=w467, f=0) -> (s? t:f=w465:i32)
                n229 = property on="字符串变量(StringVar)" class="Ring (strict)"("Value"=w465) -> ()  [unwired: 2 in, 2 out]
              }
              frame "StartWith" {
                n230 = Unbundle By Name(w487) -> ("StartWith"=w486:T20)
                n231 = call <vilib>:"Unflatten From JSON String.vi"("Type and Defaults"=w486, "error in (no error)"=w490, "JSON String"=w492) -> ("error out"=w493:errorcluster, "Variant"=w494:variant)  [unwired: 7 in]
                n232 = Variant To Data(error in=w493, type=w486, Variant=w494) -> (data=w491:T20, error out=w489:errorcluster)
                n233 = Unbundle By Name(w491) -> ("json.Method"=w488:string, "json.StringVar"=w480:string, "json.SubString"=w479:string, "json.IgnoreCasse"=w478:bool)
                n234 = property on="字符串变量(StringVar)" class="Ring (strict)"() -> ("Strings []"=w483:string[])  [unwired: 2 in, 2 out]
                n235 = local write "子字符串_StartWith"(w479) -> ()
                n236 = local write "忽略大小写_StartWith"(w478) -> ()
                n237 = Search 1D Array(1D array=w483, element=w480) -> (index of element=w485:i32)  [unwired: 1 in]
                n238 = Greater Or Equal To 0?(x=w485) -> (x >= 0?=w484:bool)
                n239 = Select(t=w485, s=w484, f=0) -> (s? t:f=w482:i32)
                n240 = property on="字符串变量(StringVar)" class="Ring (strict)"("Value"=w482) -> ()  [unwired: 2 in, 2 out]
              }
              frame "EndWith" {
                n241 = Unbundle By Name(w504) -> ("EndWith"=w503:T20)
                n242 = call <vilib>:"Unflatten From JSON String.vi"("Type and Defaults"=w503, "error in (no error)"=w507, "JSON String"=w509) -> ("error out"=w510:errorcluster, "Variant"=w511:variant)  [unwired: 7 in]
                n243 = Variant To Data(error in=w510, type=w503, Variant=w511) -> (data=w508:T20, error out=w506:errorcluster)
                n244 = Unbundle By Name(w508) -> ("json.Method"=w505:string, "json.StringVar"=w497:string, "json.SubString"=w496:string, "json.IgnoreCasse"=w495:bool)
                n245 = property on="字符串变量(StringVar)" class="Ring (strict)"() -> ("Strings []"=w500:string[])  [unwired: 2 in, 2 out]
                n246 = local write "忽略大小写_EndWith"(w495) -> ()
                n247 = local write "子字符串_EndWith"(w496) -> ()
                n248 = Search 1D Array(1D array=w500, element=w497) -> (index of element=w502:i32)  [unwired: 1 in]
                n249 = Greater Or Equal To 0?(x=w502) -> (x >= 0?=w501:bool)
                n250 = Select(t=w502, s=w501, f=0) -> (s? t:f=w499:i32)
                n251 = property on="字符串变量(StringVar)" class="Ring (strict)"("Value"=w499) -> ()  [unwired: 2 in, 2 out]
              }
              frame "AfterSubstring" {
                n252 = Unbundle By Name(w520) -> ("AfterSubstring"=w519:T21)
                n253 = call <vilib>:"Unflatten From JSON String.vi"("Type and Defaults"=w519, "error in (no error)"=w523, "JSON String"=w525) -> ("error out"=w526:errorcluster, "Variant"=w527:variant)  [unwired: 7 in]
                n254 = Variant To Data(error in=w526, type=w519, Variant=w527) -> (data=w524:T21, error out=w522:errorcluster)
                n255 = Unbundle By Name(w524) -> ("json.Method"=w521:string, "json.StringVar"=w513:string, "json.SubString"=w512:string)
                n256 = local write "SubString_AfterSubstring"(w512) -> ()
                n257 = property on="字符串变量(StringVar)" class="Ring (strict)"() -> ("Strings []"=w516:string[])  [unwired: 2 in, 2 out]
                n258 = Search 1D Array(1D array=w516, element=w513) -> (index of element=w518:i32)  [unwired: 1 in]
                n259 = Greater Or Equal To 0?(x=w518) -> (x >= 0?=w517:bool)
                n260 = Select(t=w518, s=w517, f=0) -> (s? t:f=w515:i32)
                n261 = property on="字符串变量(StringVar)" class="Ring (strict)"("Value"=w515) -> ()  [unwired: 2 in, 2 out]
              }
              frame "BeforeSubstring" {
                n262 = Unbundle By Name(w536) -> ("BeforeSubstring"=w535:T21)
                n263 = call <vilib>:"Unflatten From JSON String.vi"("Type and Defaults"=w535, "error in (no error)"=w539, "JSON String"=w541) -> ("error out"=w542:errorcluster, "Variant"=w543:variant)  [unwired: 7 in]
                n264 = Variant To Data(error in=w542, type=w535, Variant=w543) -> (data=w540:T21, error out=w538:errorcluster)
                n265 = Unbundle By Name(w540) -> ("json.Method"=w537:string, "json.StringVar"=w529:string, "json.SubString"=w528:string)
                n266 = local write "SubString_BeforeSubstring"(w528) -> ()
                n267 = property on="字符串变量(StringVar)" class="Ring (strict)"() -> ("Strings []"=w532:string[])  [unwired: 2 in, 2 out]
                n268 = Search 1D Array(1D array=w532, element=w529) -> (index of element=w534:i32)  [unwired: 1 in]
                n269 = Greater Or Equal To 0?(x=w534) -> (x >= 0?=w533:bool)
                n270 = Select(t=w534, s=w533, f=0) -> (s? t:f=w531:i32)
                n271 = property on="字符串变量(StringVar)" class="Ring (strict)"("Value"=w531) -> ()  [unwired: 2 in, 2 out]
              }
              frame "MiddleSubstring" {
                n272 = Unbundle By Name(w553) -> ("MiddleSubstring"=w552:T22)
                n273 = call <vilib>:"Unflatten From JSON String.vi"("Type and Defaults"=w552, "error in (no error)"=w556, "JSON String"=w558) -> ("error out"=w559:errorcluster, "Variant"=w560:variant)  [unwired: 7 in]
                n274 = Variant To Data(error in=w559, type=w552, Variant=w560) -> (data=w557:T22, error out=w555:errorcluster)
                n275 = Unbundle By Name(w557) -> ("json.Method"=w554:string, "json.StringVar"=w546:string, "json.BeforeSubString"=w545:string, "json.AfterSubString"=w544:string)
                n276 = property on="字符串变量(StringVar)" class="Ring (strict)"() -> ("Strings []"=w549:string[])  [unwired: 2 in, 2 out]
                n277 = local write "前子字符串_MiddleSubstring"(w545) -> ()
                n278 = local write "后子字符串_MiddleSubstring"(w544) -> ()
                n279 = Search 1D Array(1D array=w549, element=w546) -> (index of element=w551:i32)  [unwired: 1 in]
                n280 = Greater Or Equal To 0?(x=w551) -> (x >= 0?=w550:bool)
                n281 = Select(t=w551, s=w550, f=0) -> (s? t:f=w548:i32)
                n282 = property on="字符串变量(StringVar)" class="Ring (strict)"("Value"=w548) -> ()  [unwired: 2 in, 2 out]
              }
              frame "AsciiToHexString" {
                n283 = Unbundle By Name(w568) -> ("AsciiToHexString"=w567:T11)
                n284 = call <vilib>:"Unflatten From JSON String.vi"("Type and Defaults"=w567, "error in (no error)"=w571, "JSON String"=w573) -> ("error out"=w574:errorcluster, "Variant"=w575:variant)  [unwired: 7 in]
                n285 = Variant To Data(error in=w574, type=w567, Variant=w575) -> (data=w572:T11, error out=w570:errorcluster)
                n286 = Unbundle By Name(w572) -> ("json.Method"=w569:string, "json.StringVar"=w561:string)
                n287 = property on="字符串变量(StringVar)" class="Ring (strict)"() -> ("Strings []"=w564:string[])  [unwired: 2 in, 2 out]
                n288 = Search 1D Array(1D array=w564, element=w561) -> (index of element=w566:i32)  [unwired: 1 in]
                n289 = Greater Or Equal To 0?(x=w566) -> (x >= 0?=w565:bool)
                n290 = Select(t=w566, s=w565, f=0) -> (s? t:f=w563:i32)
                n291 = property on="字符串变量(StringVar)" class="Ring (strict)"("Value"=w563) -> ()  [unwired: 2 in, 2 out]
              }
              frame "HexStringToAscii" {
                n292 = Unbundle By Name(w583) -> ("HexStringToAscii"=w582:T11)
                n293 = call <vilib>:"Unflatten From JSON String.vi"("Type and Defaults"=w582, "error in (no error)"=w586, "JSON String"=w588) -> ("error out"=w589:errorcluster, "Variant"=w590:variant)  [unwired: 7 in]
                n294 = Variant To Data(error in=w589, type=w582, Variant=w590) -> (data=w587:T11, error out=w585:errorcluster)
                n295 = Unbundle By Name(w587) -> ("json.Method"=w584:string, "json.StringVar"=w576:string)
                n296 = property on="字符串变量(StringVar)" class="Ring (strict)"() -> ("Strings []"=w579:string[])  [unwired: 2 in, 2 out]
                n297 = Search 1D Array(1D array=w579, element=w576) -> (index of element=w581:i32)  [unwired: 1 in]
                n298 = Greater Or Equal To 0?(x=w581) -> (x >= 0?=w580:bool)
                n299 = Select(t=w581, s=w580, f=0) -> (s? t:f=w578:i32)
                n300 = property on="字符串变量(StringVar)" class="Ring (strict)"("Value"=w578) -> ()  [unwired: 2 in, 2 out]
              }
              frame "StringTo1DArray" {
                n301 = Unbundle By Name(w599) -> ("StringTo1DArray"=w598:T23)
                n302 = call <vilib>:"Unflatten From JSON String.vi"("Type and Defaults"=w598, "error in (no error)"=w602, "JSON String"=w604) -> ("error out"=w605:errorcluster, "Variant"=w606:variant)  [unwired: 7 in]
                n303 = Variant To Data(error in=w605, type=w598, Variant=w606) -> (data=w603:T23, error out=w601:errorcluster)
                n304 = Unbundle By Name(w603) -> ("json.Method"=w600:string, "json.StringVar"=w592:string, "json.Delimiter"=w591:string)
                n305 = local write "Delimiter_StringTo1DArray"(w591) -> ()
                n306 = property on="字符串变量(StringVar)" class="Ring (strict)"() -> ("Strings []"=w595:string[])  [unwired: 2 in, 2 out]
                n307 = Search 1D Array(1D array=w595, element=w592) -> (index of element=w597:i32)  [unwired: 1 in]
                n308 = Greater Or Equal To 0?(x=w597) -> (x >= 0?=w596:bool)
                n309 = Select(t=w597, s=w596, f=0) -> (s? t:f=w594:i32)
                n310 = property on="字符串变量(StringVar)" class="Ring (strict)"("Value"=w594) -> ()  [unwired: 2 in, 2 out]
              }
              frame "StringToCharacterArray" {
                n311 = Unbundle By Name(w614) -> ("StringToCharacterArray"=w613:T11)
                n312 = call <vilib>:"Unflatten From JSON String.vi"("Type and Defaults"=w613, "error in (no error)"=w617, "JSON String"=w619) -> ("error out"=w620:errorcluster, "Variant"=w621:variant)  [unwired: 7 in]
                n313 = Variant To Data(error in=w620, type=w613, Variant=w621) -> (data=w618:T11, error out=w616:errorcluster)
                n314 = Unbundle By Name(w618) -> ("json.Method"=w615:string, "json.StringVar"=w607:string)
                n315 = property on="字符串变量(StringVar)" class="Ring (strict)"() -> ("Strings []"=w610:string[])  [unwired: 2 in, 2 out]
                n316 = Search 1D Array(1D array=w610, element=w607) -> (index of element=w612:i32)  [unwired: 1 in]
                n317 = Greater Or Equal To 0?(x=w612) -> (x >= 0?=w611:bool)
                n318 = Select(t=w612, s=w611, f=0) -> (s? t:f=w609:i32)
                n319 = property on="字符串变量(StringVar)" class="Ring (strict)"("Value"=w609) -> ()  [unwired: 2 in, 2 out]
              }
              frame "RemoveAllWhitespace" {
                n320 = Unbundle By Name(w629) -> ("RemoveAllWhitespace"=w628:T11)
                n321 = call <vilib>:"Unflatten From JSON String.vi"("Type and Defaults"=w628, "error in (no error)"=w632, "JSON String"=w634) -> ("error out"=w635:errorcluster, "Variant"=w636:variant)  [unwired: 7 in]
                n322 = Variant To Data(error in=w635, type=w628, Variant=w636) -> (data=w633:T11, error out=w631:errorcluster)
                n323 = Unbundle By Name(w633) -> ("json.Method"=w630:string, "json.StringVar"=w622:string)
                n324 = property on="字符串变量(StringVar)" class="Ring (strict)"() -> ("Strings []"=w625:string[])  [unwired: 2 in, 2 out]
                n325 = Search 1D Array(1D array=w625, element=w622) -> (index of element=w627:i32)  [unwired: 1 in]
                n326 = Greater Or Equal To 0?(x=w627) -> (x >= 0?=w626:bool)
                n327 = Select(t=w627, s=w626, f=0) -> (s? t:f=w624:i32)
                n328 = property on="字符串变量(StringVar)" class="Ring (strict)"("Value"=w624) -> ()  [unwired: 2 in, 2 out]
              }
              frame Default {
              }
            }
            n329 = property on="方法(Method)" class="Enum (strict)"() -> ("Strings []"=w244:string[])  [unwired: 2 in, 2 out]
            n330 = Search 1D Array(1D array=w244, element=w242) -> (index of element=w246:i32)  [unwired: 1 in]
            n331 = Greater Or Equal To 0?(x=w246) -> (x >= 0?=w245:bool)
            n332 = Select(t=w246, s=w245, f=0) -> (s? t:f=w241:i32)
            n333 = local write "ArrayType"(w241) -> ()
            n334 = property on="方法(Method)" class="Enum (strict)"("Value"=w241) -> ()  [unwired: 2 in, 2 out]
          }
          frame True {
          }
        }
        n335 = call <vilib>:"Add State(s) to Queue__JKI_lib_State_Machine.vi"("State(s) in (\"\")"=w240) -> ("States Out"=w239:string)  [unwired: 14 in]
      }
      frame "Parameter: Combin Parameter" {
        n336 = property on="方法(Method)" class="Enum (strict)"() -> ("RingText.Text"=w642:string)  [unwired: 2 in, 2 out]
        n337 = Unbundle By Name(w640) -> ("StringClusters"=w639:T5)
        n338 = case shown="\"StringTo1DArray\"" w642 {
          selector: w642 -> [_ w650 w660 w671 w681 w693 w707 w718 w731 w740 w749 w758 w767 w776 w785 w796 w807 w817 w827 w838 w847 w856 w866 w875 w884]
          tunnel: w639 -> [_ w657 w666 w677 w687 w699 w713 w724 w737 w747 w756 w765 w774 w783 w792 w803 w814 w824 w834 w845 w854 w863 w873 w882 w891]
          tunnel: [_ w655 w664 w675 w685 w697 w711 w722 w735 w745 w754 w763 w772 w781 w790 w801 w812 w822 w832 w843 w852 w861 w871 w880 w889] -> w641
          tunnel: [w648 w649 w659 w670 w680 w692 w706 w717 w730 w741 w750 w759 w768 w777 w786 w797 w808 w818 w828 w839 w848 w857 w867 w876 w885] -> w644
          tunnel: w643 -> [w648 w653 w662 w673 w683 w695 w709 w720 w733 w743 w752 w761 w770 w779 w788 w799 w810 w820 w830 w841 w850 w859 w869 w878 w887]
          frame Default {
          }
          frame "StringLength" {
            n339 = property on="字符串变量(StringVar)" class="Ring (strict)"() -> ("RingText.Text"=w652:string)  [unwired: 2 in, 2 out]
            n340 = Unbundle By Name(w657) -> ("StringLength"=w656:T11)
            n341 = Bundle By Name(cluster=w656, "json.Method"=w650, "json.StringVar"=w652) -> (w651:T11)
            n342 = call <vilib>:"Flatten To JSON String.vi"("Multiline (T)"=TRUE, "error in (no error)"=w653, "Variant"=w651) -> ("error out"=w649:errorcluster, "JSON String"=w655:string)  [unwired: 7 in]
          }
          frame "InitialString" {
            n343 = local read "字符串_InitialString"() -> (w658:string)
            n344 = Unbundle By Name(w666) -> ("InitialString"=w665:T12)
            n345 = Bundle By Name(cluster=w665, "json.Method"=w660, "json.Strings"=w658) -> (w661:T12)
            n346 = call <vilib>:"Flatten To JSON String.vi"("Multiline (T)"=TRUE, "error in (no error)"=w662, "Variant"=w661) -> ("error out"=w659:errorcluster, "JSON String"=w664:string)  [unwired: 7 in]
          }
          frame "StringSubset" {
            n347 = local read "偏移_StringSubset"() -> (w668:i32)
            n348 = local read "长度_StringSubset"() -> (w667:i32)
            n349 = property on="字符串变量(StringVar)" class="Ring (strict)"() -> ("RingText.Text"=w669:string)  [unwired: 2 in, 2 out]
            n350 = Unbundle By Name(w677) -> ("StringSubset"=w676:T13)
            n351 = Bundle By Name(cluster=w676, "json.Method"=w671, "json.StringVar"=w669, "json.offset"=w668, "json.length"=w667) -> (w672:T13)
            n352 = call <vilib>:"Flatten To JSON String.vi"("Multiline (T)"=TRUE, "error in (no error)"=w673, "Variant"=w672) -> ("error out"=w670:errorcluster, "JSON String"=w675:string)  [unwired: 7 in]
          }
          frame "TrimWhitespace" {
            n353 = property on="字符串变量(StringVar)" class="Ring (strict)"() -> ("RingText.Text"=w679:string)  [unwired: 2 in, 2 out]
            n354 = property on="位置_TrimWhitespace" class="Ring (strict)"() -> ("RingText.Text"=w678:string)  [unwired: 2 in, 2 out]
            n355 = Unbundle By Name(w687) -> ("TrimWhitespace"=w686:T14)
            n356 = Bundle By Name(cluster=w686, "json.Method"=w681, "json.StringVar"=w679, "json.Location"=w678) -> (w682:T14)
            n357 = call <vilib>:"Flatten To JSON String.vi"("Multiline (T)"=TRUE, "error in (no error)"=w683, "Variant"=w682) -> ("error out"=w680:errorcluster, "JSON String"=w685:string)  [unwired: 7 in]
          }
          frame "ReplaceSubstring" {
            n358 = local read "偏移_ReplaceSubstring"() -> (w689:i32)
            n359 = local read "子字符串_ReplaceSubstring"() -> (w690:string)
            n360 = local read "长度_ReplaceSubstring"() -> (w688:i32)
            n361 = property on="字符串变量(StringVar)" class="Ring (strict)"() -> ("RingText.Text"=w691:string)  [unwired: 2 in, 2 out]
            n362 = Unbundle By Name(w699) -> ("ReplaceSubstring"=w698:T15)
            n363 = Bundle By Name(cluster=w698, "json.Method"=w693, "json.StringVar"=w691, "json.Substring"=w690, "json.Offset"=w689, "json.Length"=w688) -> (w694:T15)
            n364 = call <vilib>:"Flatten To JSON String.vi"("Multiline (T)"=TRUE, "error in (no error)"=w695, "Variant"=w694) -> ("error out"=w692:errorcluster, "JSON String"=w697:string)  [unwired: 7 in]
          }
          frame "SearchandReplaceString" {
            n365 = local read "IgnoreCase_SearchandReplaceString"() -> (w700:bool)
            n366 = local read "ReplaceAll_SearchandReplaceString"() -> (w701:bool)
            n367 = local read "搜索字符串_SearchandReplaceString"() -> (w703:string)
            n368 = local read "替换字符串_SearchandReplaceString"() -> (w702:string)
            n369 = local read "偏移_SearchandReplaceString"() -> (w704:i32)
            n370 = property on="字符串变量(StringVar)" class="Ring (strict)"() -> ("RingText.Text"=w705:string)  [unwired: 2 in, 2 out]
            n371 = Unbundle By Name(w713) -> ("SearchandReplaceString"=w712:T16)
            n372 = Bundle By Name(cluster=w712, "json.Method"=w707, "json.StringVar"=w705, "json.SearchString"=w703, "json.Offset"=w704, "json.ReplaceString"=w702, "json.ReplaceAll"=w701, "json.IgnoreCase"=w700) -> (w708:T16)
            n373 = call <vilib>:"Flatten To JSON String.vi"("Multiline (T)"=TRUE, "error in (no error)"=w709, "Variant"=w708) -> ("error out"=w706:errorcluster, "JSON String"=w711:string)  [unwired: 7 in]
          }
          frame "MatchPattern" {
            n374 = local read "正则表达式_MatchPattern"() -> (w715:string)
            n375 = local read "偏移_MatchPattern"() -> (w714:i32)
            n376 = property on="字符串变量(StringVar)" class="Ring (strict)"() -> ("RingText.Text"=w716:string)  [unwired: 2 in, 2 out]
            n377 = Unbundle By Name(w724) -> ("MatchPattern"=w723:T17)
            n378 = Bundle By Name(cluster=w723, "json.Method"=w718, "json.StringVar"=w716, "json.RegularExpression"=w715, "json.Offset"=w714) -> (w719:T17)
            n379 = call <vilib>:"Flatten To JSON String.vi"("Multiline (T)"=TRUE, "error in (no error)"=w720, "Variant"=w719) -> ("error out"=w717:errorcluster, "JSON String"=w722:string)  [unwired: 7 in]
          }
          frame "MatchRegularExpression" {
            n380 = local read "正则表达式_MatchRegularExpression"() -> (w728:string)
            n381 = local read "偏移_MatchRegularExpression"() -> (w727:i32)
            n382 = local read "忽略大小写_MatchRegularExpression"() -> (w726:bool)
            n383 = local read "多行_MatchRegularExpression"() -> (w725:bool)
            n384 = property on="字符串变量(StringVar)" class="Ring (strict)"() -> ("RingText.Text"=w729:string)  [unwired: 2 in, 2 out]
            n385 = Unbundle By Name(w737) -> ("MatchRegularExpression"=w736:T18)
            n386 = Bundle By Name(cluster=w736, "json.Method"=w731, "json.StringVar"=w729, "json.RegularExpression"=w728, "json.Offset"=w727, "json.IgnoreCase"=w726, "json.Multiline"=w725) -> (w732:T18)
            n387 = call <vilib>:"Flatten To JSON String.vi"("Multiline (T)"=TRUE, "error in (no error)"=w733, "Variant"=w732) -> ("error out"=w730:errorcluster, "JSON String"=w735:string)  [unwired: 7 in]
          }
          frame "FormatDate/TimeString" {
            n388 = local read "时间格式字符串_FormatDate/TimeString"() -> (w739:string)
            n389 = local read "UTC格式_FormatDate/TimeString"() -> (w738:bool)
            n390 = Unbundle By Name(w747) -> ("FormatDate/TimeString"=w746:T19)
            n391 = Bundle By Name(cluster=w746, "json.Method"=w740, "json.TimeFormatString"=w739, "json.UTCFormat"=w738) -> (w742:T19)
            n392 = call <vilib>:"Flatten To JSON String.vi"("Multiline (T)"=TRUE, "error in (no error)"=w743, "Variant"=w742) -> ("error out"=w741:errorcluster, "JSON String"=w745:string)  [unwired: 7 in]
          }
          frame "ToLowerCase" {
            n393 = property on="字符串变量(StringVar)" class="Ring (strict)"() -> ("RingText.Text"=w748:string)  [unwired: 2 in, 2 out]
            n394 = Unbundle By Name(w756) -> ("ToLowerCase"=w755:T11)
            n395 = Bundle By Name(cluster=w755, "json.Method"=w749, "json.StringVar"=w748) -> (w751:T11)
            n396 = call <vilib>:"Flatten To JSON String.vi"("Multiline (T)"=TRUE, "error in (no error)"=w752, "Variant"=w751) -> ("error out"=w750:errorcluster, "JSON String"=w754:string)  [unwired: 7 in]
          }
          frame "ToUpperCase" {
            n397 = property on="字符串变量(StringVar)" class="Ring (strict)"() -> ("RingText.Text"=w757:string)  [unwired: 2 in, 2 out]
            n398 = Unbundle By Name(w765) -> ("ToUpperCase"=w764:T11)
            n399 = Bundle By Name(cluster=w764, "json.Method"=w758, "json.StringVar"=w757) -> (w760:T11)
            n400 = call <vilib>:"Flatten To JSON String.vi"("Multiline (T)"=TRUE, "error in (no error)"=w761, "Variant"=w760) -> ("error out"=w759:errorcluster, "JSON String"=w763:string)  [unwired: 7 in]
          }
          frame "StringMD5" {
            n401 = property on="字符串变量(StringVar)" class="Ring (strict)"() -> ("RingText.Text"=w766:string)  [unwired: 2 in, 2 out]
            n402 = Unbundle By Name(w774) -> ("StringMD5"=w773:T11)
            n403 = Bundle By Name(cluster=w773, "json.Method"=w767, "json.StringVar"=w766) -> (w769:T11)
            n404 = call <vilib>:"Flatten To JSON String.vi"("Multiline (T)"=TRUE, "error in (no error)"=w770, "Variant"=w769) -> ("error out"=w768:errorcluster, "JSON String"=w772:string)  [unwired: 7 in]
          }
          frame "NumStringToHexString" {
            n405 = property on="字符串变量(StringVar)" class="Ring (strict)"() -> ("RingText.Text"=w775:string)  [unwired: 2 in, 2 out]
            n406 = Unbundle By Name(w783) -> ("NumStringToHexString"=w782:T11)
            n407 = Bundle By Name(cluster=w782, "json.Method"=w776, "json.StringVar"=w775) -> (w778:T11)
            n408 = call <vilib>:"Flatten To JSON String.vi"("Multiline (T)"=TRUE, "error in (no error)"=w779, "Variant"=w778) -> ("error out"=w777:errorcluster, "JSON String"=w781:string)  [unwired: 7 in]
          }
          frame "HexStringToNumString" {
            n409 = property on="字符串变量(StringVar)" class="Ring (strict)"() -> ("RingText.Text"=w784:string)  [unwired: 2 in, 2 out]
            n410 = Unbundle By Name(w792) -> ("HexStringToNumString"=w791:T11)
            n411 = Bundle By Name(cluster=w791, "json.Method"=w785, "json.StringVar"=w784) -> (w787:T11)
            n412 = call <vilib>:"Flatten To JSON String.vi"("Multiline (T)"=TRUE, "error in (no error)"=w788, "Variant"=w787) -> ("error out"=w786:errorcluster, "JSON String"=w790:string)  [unwired: 7 in]
          }
          frame "StartWith" {
            n413 = local read "忽略大小写_StartWith"() -> (w793:bool)
            n414 = local read "子字符串_StartWith"() -> (w794:string)
            n415 = property on="字符串变量(StringVar)" class="Ring (strict)"() -> ("RingText.Text"=w795:string)  [unwired: 2 in, 2 out]
            n416 = Unbundle By Name(w803) -> ("StartWith"=w802:T20)
            n417 = Bundle By Name(cluster=w802, "json.Method"=w796, "json.StringVar"=w795, "json.SubString"=w794, "json.IgnoreCasse"=w793) -> (w798:T20)
            n418 = call <vilib>:"Flatten To JSON String.vi"("Multiline (T)"=TRUE, "error in (no error)"=w799, "Variant"=w798) -> ("error out"=w797:errorcluster, "JSON String"=w801:string)  [unwired: 7 in]
          }
          frame "EndWith" {
            n419 = local read "子字符串_EndWith"() -> (w805:string)
            n420 = local read "忽略大小写_EndWith"() -> (w804:bool)
            n421 = property on="字符串变量(StringVar)" class="Ring (strict)"() -> ("RingText.Text"=w806:string)  [unwired: 2 in, 2 out]
            n422 = Unbundle By Name(w814) -> ("EndWith"=w813:T20)
            n423 = Bundle By Name(cluster=w813, "json.Method"=w807, "json.StringVar"=w806, "json.SubString"=w805, "json.IgnoreCasse"=w804) -> (w809:T20)
            n424 = call <vilib>:"Flatten To JSON String.vi"("Multiline (T)"=TRUE, "error in (no error)"=w810, "Variant"=w809) -> ("error out"=w808:errorcluster, "JSON String"=w812:string)  [unwired: 7 in]
          }
          frame "AfterSubstring" {
            n425 = local read "SubString_AfterSubstring"() -> (w815:string)
            n426 = property on="字符串变量(StringVar)" class="Ring (strict)"() -> ("RingText.Text"=w816:string)  [unwired: 2 in, 2 out]
            n427 = Unbundle By Name(w824) -> ("AfterSubstring"=w823:T21)
            n428 = Bundle By Name(cluster=w823, "json.Method"=w817, "json.StringVar"=w816, "json.SubString"=w815) -> (w819:T21)
            n429 = call <vilib>:"Flatten To JSON String.vi"("Multiline (T)"=TRUE, "error in (no error)"=w820, "Variant"=w819) -> ("error out"=w818:errorcluster, "JSON String"=w822:string)  [unwired: 7 in]
          }
          frame "BeforeSubstring" {
            n430 = local read "SubString_BeforeSubstring"() -> (w825:string)
            n431 = property on="字符串变量(StringVar)" class="Ring (strict)"() -> ("RingText.Text"=w826:string)  [unwired: 2 in, 2 out]
            n432 = Unbundle By Name(w834) -> ("BeforeSubstring"=w833:T21)
            n433 = Bundle By Name(cluster=w833, "json.Method"=w827, "json.StringVar"=w826, "json.SubString"=w825) -> (w829:T21)
            n434 = call <vilib>:"Flatten To JSON String.vi"("Multiline (T)"=TRUE, "error in (no error)"=w830, "Variant"=w829) -> ("error out"=w828:errorcluster, "JSON String"=w832:string)  [unwired: 7 in]
          }
          frame "MiddleSubstring" {
            n435 = local read "前子字符串_MiddleSubstring"() -> (w836:string)
            n436 = local read "后子字符串_MiddleSubstring"() -> (w835:string)
            n437 = property on="字符串变量(StringVar)" class="Ring (strict)"() -> ("RingText.Text"=w837:string)  [unwired: 2 in, 2 out]
            n438 = Unbundle By Name(w845) -> ("MiddleSubstring"=w844:T22)
            n439 = Bundle By Name(cluster=w844, "json.Method"=w838, "json.StringVar"=w837, "json.BeforeSubString"=w836, "json.AfterSubString"=w835) -> (w840:T22)
            n440 = call <vilib>:"Flatten To JSON String.vi"("Multiline (T)"=TRUE, "error in (no error)"=w841, "Variant"=w840) -> ("error out"=w839:errorcluster, "JSON String"=w843:string)  [unwired: 7 in]
          }
          frame "AsciiToHexString" {
            n441 = property on="字符串变量(StringVar)" class="Ring (strict)"() -> ("RingText.Text"=w846:string)  [unwired: 2 in, 2 out]
            n442 = Unbundle By Name(w854) -> ("AsciiToHexString"=w853:T11)
            n443 = Bundle By Name(cluster=w853, "json.Method"=w847, "json.StringVar"=w846) -> (w849:T11)
            n444 = call <vilib>:"Flatten To JSON String.vi"("Multiline (T)"=TRUE, "error in (no error)"=w850, "Variant"=w849) -> ("error out"=w848:errorcluster, "JSON String"=w852:string)  [unwired: 7 in]
          }
          frame "HexStringToAscii" {
            n445 = property on="字符串变量(StringVar)" class="Ring (strict)"() -> ("RingText.Text"=w855:string)  [unwired: 2 in, 2 out]
            n446 = Unbundle By Name(w863) -> ("HexStringToAscii"=w862:T11)
            n447 = Bundle By Name(cluster=w862, "json.Method"=w856, "json.StringVar"=w855) -> (w858:T11)
            n448 = call <vilib>:"Flatten To JSON String.vi"("Multiline (T)"=TRUE, "error in (no error)"=w859, "Variant"=w858) -> ("error out"=w857:errorcluster, "JSON String"=w861:string)  [unwired: 7 in]
          }
          frame "StringTo1DArray" {
            n449 = local read "Delimiter_StringTo1DArray"() -> (w864:string)
            n450 = property on="字符串变量(StringVar)" class="Ring (strict)"() -> ("RingText.Text"=w865:string)  [unwired: 2 in, 2 out]
            n451 = Unbundle By Name(w873) -> ("StringTo1DArray"=w872:T23)
            n452 = Bundle By Name(cluster=w872, "json.Method"=w866, "json.StringVar"=w865, "json.Delimiter"=w864) -> (w868:T23)
            n453 = call <vilib>:"Flatten To JSON String.vi"("Multiline (T)"=TRUE, "error in (no error)"=w869, "Variant"=w868) -> ("error out"=w867:errorcluster, "JSON String"=w871:string)  [unwired: 7 in]
          }
          frame "StringToCharacterArray" {
            n454 = property on="字符串变量(StringVar)" class="Ring (strict)"() -> ("RingText.Text"=w874:string)  [unwired: 2 in, 2 out]
            n455 = Unbundle By Name(w882) -> ("StringToCharacterArray"=w881:T11)
            n456 = Bundle By Name(cluster=w881, "json.Method"=w875, "json.StringVar"=w874) -> (w877:T11)
            n457 = call <vilib>:"Flatten To JSON String.vi"("Multiline (T)"=TRUE, "error in (no error)"=w878, "Variant"=w877) -> ("error out"=w876:errorcluster, "JSON String"=w880:string)  [unwired: 7 in]
          }
          frame "RemoveAllWhitespace" {
            n458 = property on="字符串变量(StringVar)" class="Ring (strict)"() -> ("RingText.Text"=w883:string)  [unwired: 2 in, 2 out]
            n459 = Unbundle By Name(w891) -> ("RemoveAllWhitespace"=w890:T11)
            n460 = Bundle By Name(cluster=w890, "json.Method"=w884, "json.StringVar"=w883) -> (w886:T11)
            n461 = call <vilib>:"Flatten To JSON String.vi"("Multiline (T)"=TRUE, "error in (no error)"=w887, "Variant"=w886) -> ("error out"=w885:errorcluster, "JSON String"=w889:string)  [unwired: 7 in]
          }
        }
        n462 = Bundle By Name(cluster=w640, "Synchronize.Echo.JsonOut"=w641) -> (w645:T8)
        n463 = call <vilib>:"Add State(s) to Queue__JKI_lib_State_Machine.vi"("State(s) in (\"\")"=w647) -> ("States Out"=w646:string)  [unwired: 14 in]
      }
      frame "---------- Sync ----------" {
        n464 = call <vilib>:"Add State(s) to Queue__JKI_lib_State_Machine.vi"("State(s) in (\"\")"=w895) -> ("States Out"=w894:string)  [unwired: 14 in]
      }
      frame "Sync: Obtain CMD Queue" {
        # "这里由平台输入"
        n465 = Unbundle By Name(w897) -> ("Synchronize.EnqueueData"=w896:T24)
        n466 = Obtain Queue(name (unnamed)="VIId", element data type=w896, error in (no error)=w902) -> (queue out=w898:refnum<queue>, error out=w901:errorcluster)  [unwired: 2 in, 1 out]
        n467 = Bundle By Name(cluster=w897, "Synchronize.Queue"=w898) -> (w899:T8)
        n468 = call <vilib>:"Add State(s) to Queue__JKI_lib_State_Machine.vi"("State(s) in (\"\")"=w904) -> ("States Out"=w903:string)  [unwired: 14 in]
      }
      frame "Sync: Dequeue CMD" {
        n469 = Unbundle By Name(w917) -> ("Synchronize.Queue"=w914:refnum<queue>, "Synchronize.Communicate"=w905:T25)
        n470 = Dequeue Element(queue=w914, timeout in ms (-1)=10, error in (no error)=w915) -> (queue out=w913:refnum<queue>, element=w911:T24, timed out?=w912:bool, error out=w907:errorcluster)
        n471 = Bundle By Name(cluster=w917, "Synchronize.Queue"=w913, "Synchronize.EnqueueData"=w911) -> (w909:T8)
        n472 = case shown="False" w912 {
          tunnel: w911 -> [w928 _]
          tunnel: [w926 _] -> w910
          tunnel: w909 -> [w925 w957]
          tunnel: [w924 w957] -> w908
          tunnel: w907 -> [w922 w956]
          tunnel: [w921 w956] -> w906
          tunnel: w905 -> [w920 _]
          frame False {
            n473 = Unbundle By Name(w928) -> ("Action"=w927:T26, "Data"=w923:variant)
            n474 = case shown="\"Query\"" w927 {
              tunnel: ["Sync: Send ECHO" "UI: Initialize VarList\nSync: Send ECHO" _ "Sync: Send ECHO\nMacro: Exit" "Parameter: Combin Parameter\nSync: Send ECHO" "Parameter: Parse Parameter\nSync: Send ECHO"] -> w926
              tunnel: w925 -> [w931 w936 w940 w943 w948 w953]
              tunnel: [w930 w935 w940 w942 w947 w952] -> w924
              tunnel: w923 -> [_ _ _ _ _ _]
              tunnel: w922 -> [w932 w937 w939 w944 w949 w954]
              tunnel: [w932 w937 w939 w944 w949 w954] -> w921
              tunnel: w920 -> [_ _ _ _ _ _]
              frame "Create" {
                n475 = Bundle By Name(cluster=w931, "Synchronize.Echo.Status"="Create Success") -> (w930:T8)
              }
              frame "UpdateVariable" {
                n476 = Bundle By Name(cluster=w936, "Synchronize.Echo.Status"="UpdateVariable Success") -> (w935:T8)
              }
              frame Default {
              }
              frame "Close" {
                n477 = Bundle By Name(cluster=w943, "Synchronize.Echo.Status"="Close Success") -> (w942:T8)
              }
              frame "Query" {
                n478 = Bundle By Name(cluster=w948, "Synchronize.Echo.Status"="Query Success") -> (w947:T8)
              }
              frame "Revert" {
                n479 = Bundle By Name(cluster=w953, "Synchronize.Echo.Status"="Revert Success") -> (w952:T8)
              }
            }
          }
          frame True {
          }
        }
        n480 = call <vilib>:"Add State(s) to Queue__JKI_lib_State_Machine.vi"("State(s) in Front (\"\")"=w910, "State(s) in (\"\")"=w919) -> ("States Out"=w918:string)  [unwired: 13 in]
      }
      frame "Sync: Release CMD Queue" {
        n481 = Unbundle By Name(w960) -> ("Synchronize.Queue"=w961:refnum<queue>)
        n482 = Release Queue(queue=w961, error in (no error)=w959) -> (error out=w958:errorcluster)  [unwired: 1 in, 2 out]
        n483 = call <vilib>:"Add State(s) to Queue__JKI_lib_State_Machine.vi"("State(s) in (\"\")"=w963) -> ("States Out"=w962:string)  [unwired: 14 in]
      }
      frame "Sync: Send ECHO" {
        n484 = Unbundle By Name(w967) -> ("Synchronize.Communicate"=w964:T25, "Synchronize.EnqueueData.Data"=w976:variant, "Synchronize.Echo"=w968:T27)
        n485 = Variant To Data(error in=w966, type=w964, Variant=w976) -> (data=w969:T25, error out=w970:errorcluster)
        n486 = Unbundle By Name(w969) -> ("ID"=w973:string)
        n487 = Obtain Queue(name (unnamed)=w973, element data type=w968, error in (no error)=w970) -> (queue out=w972:refnum<queue>, error out=w974:errorcluster)  [unwired: 2 in, 1 out]
        n488 = Enqueue Element(queue=w972, element=w968, error in (no error)=w974) -> (queue out=w971:refnum<queue>, error out=w975:errorcluster)  [unwired: 1 in, 1 out]
        n489 = Release Queue(queue=w971, error in (no error)=w975) -> (error out=w965:errorcluster)  [unwired: 1 in, 2 out]
        n490 = call <vilib>:"Add State(s) to Queue__JKI_lib_State_Machine.vi"("State(s) in (\"\")"=w978) -> ("States Out"=w977:string)  [unwired: 14 in]
      }
    }
  }
  n491 = flat-sequence {
    frame #0 {
    }
  }
